vi "Auto_New.vi"() -> ()   [LabVIEW 2017]
uses:
  Control/Saurabh/prosucer_consumer_enum1.ctl
  <vilib>/Utility/error.llb/DialogType.ctl
  <vilib>/addons/database/Connection.llb/DB Tools Open Connec (String).vi
  Global/DATA LOG.vi
  Global/Global 1.vi
  <vilib>/addons/database/NI_Database_API.lvlib
panel:
  out "SHIFT":string
  in  "BARCODE RECIPE":string(combo)
  out "PLC COM.":bool
  out "SHIFT_DATA":string[](array[string])
  out "stop":bool
  out "error out 2":errorcluster
  out "Shift 4":i32
  out "Time Stamp Out":timestamp[](array[timestamp]) format="%<%X>T"
  out "Time Stamp Out 4":timestamp[](array[timestamp]) format="%<%X>T"
  out "Shift_change":bool
  out "appended array":string[][](array[string])
  out "SHIFT_DATA 2":string[](array[string])
  in  "error in (no error)":errorcluster
  in  "Tab Control":enum32{"Screen 1", "Screen 2", "Daignostic"}(tab)
  out "OP 50":bool
  out "OP 40":bool
  out "OP 30":bool
  out "OP - 50":T1 {"RH Motor Screw" format="%#.2g N-m"; "LH Motor Screw" format="%#.2g N-m"; "Nut Torque" format="%#.2g N-m"}
  out "OP - 40":T2 {"Stack Load" format="%.2f kg"; "Dispalcement" format="%#.2g mm"; "LH Screw" format="%#.2g N-m"; "RH Screw" format="%#.2g N-m"}
  out "OP - 30":T3 {"Shaft Press Load" format="%#.2g kg"; "Displacement" format="%#.2g mm"}
  in  "stop 2":bool
  out "OP - 10":T4 {"Leak Rate" format="%#.2g SCCM"}
  in  "SIMULATE INPUT":bool[](array[boolean])=[FALSE, FALSE, FALSE, FALSE]
  out "OP - 20":T5 {"Top Load" format="%#.2g kg"; "Top Displace" format="%#.2g mm"; "Bottom Load" format="%#.2g kg"; "Bottom Displace" format="%#.2g mm"}
  out "OP 10 & 20":bool
  out "OP - 60":T6 {"Screw 6" format="%#.2g N-m"; "Screw 5" format="%#.2g N-m"; "Screw 4" format="%#.2g N-m"; "Screw 3" format="%#.2g N-m"; "Screw 2" format="%#.2g N-m"; "Screw 1" format="%#.2g N-m"}
  out "OP - 70":T7 {"Full Open" format="%#.4g V"; "Full Close" format="%#.4g V"}
  out "OP - 110":cluster{"BARCODE":string}
  out "OP - 80":T8 {"Plug Press Load" format="%#.2f kg"}
  out "OP - 90":T9 {"Steam Leak" format="%#_g sccm"; "Seat Leak" format="%#_g LPM"}
  out "OP - 100":T10 {"Response Time REV" format="%#_g msec"; "Response time FWD" format="%#_g msec"; "Motor Full Open" format="%#.2f V"; "Motor Start Back" format="%#.2f V"; "Motor Full Close" format="%#.2f V"; "Motor Start Of Close" format="%#.2f V"; "Motor Peak" format="%#.2f A"; "Sensor O/P Full Close" format="%#.2f V"; "Sensor O/P Start Of Close" format="%#.2f V"; "Sensor O/P Open" format="%#.2f V"}
  out "OP 60":bool
  out "OP 70 & 80":bool
  out "OP 90 -100 - 110":bool
  out "OP110 STATUS":dbl[](array[numeric])
  out "SCAN OP110":string[](array[string])
  out "OP100 STATUS":dbl[](array[numeric])
  out "SCAN OP100":string[](array[string])
  out "OP50 STATUS":dbl[](array[numeric])
  out "SCAN OP50":string[](array[string])
  out "OP90 STATUS":dbl[](array[numeric])
  out "SCAN OP90":string[](array[string])
  out "OP80 STATUS":dbl[](array[numeric])
  out "SCAN OP80":string[](array[string])
  out "OP70 STATUS":dbl[](array[numeric])
  out "SCAN OP70":string[](array[string])
  out "OP60 STATUS":dbl[](array[numeric])
  out "SCAN OP60":string[](array[string])
  out "OP40 STATUS":dbl[](array[numeric])
  out "SCAN OP40":string[](array[string])
  out "OP30 STATUS":dbl[](array[numeric])
  out "SCAN OP30":string[](array[string])
  out "OP20 STATUS":dbl[](array[numeric])
  out "SCAN OP20":string[](array[string])
  out "OP10 STATUS":dbl[](array[numeric])
  out "SCAN OP10":string[](array[string])
  # "Op10 20\nOp30\nOp 40\nOp50\nOp60\nOp70-80\nOp 90-100-110"
  # "SENSOR MIN VLTG"
  # "OP - 50"
  # "OP - 40"
  # "OP - 30"
  # "OP - 10"
  # "OP - 20"
  # "OP - 60"
  # "OP - 70"
  # "OP - 110"
  # "OP - 80"
  # "OP - 90"
  # "OP - 100"
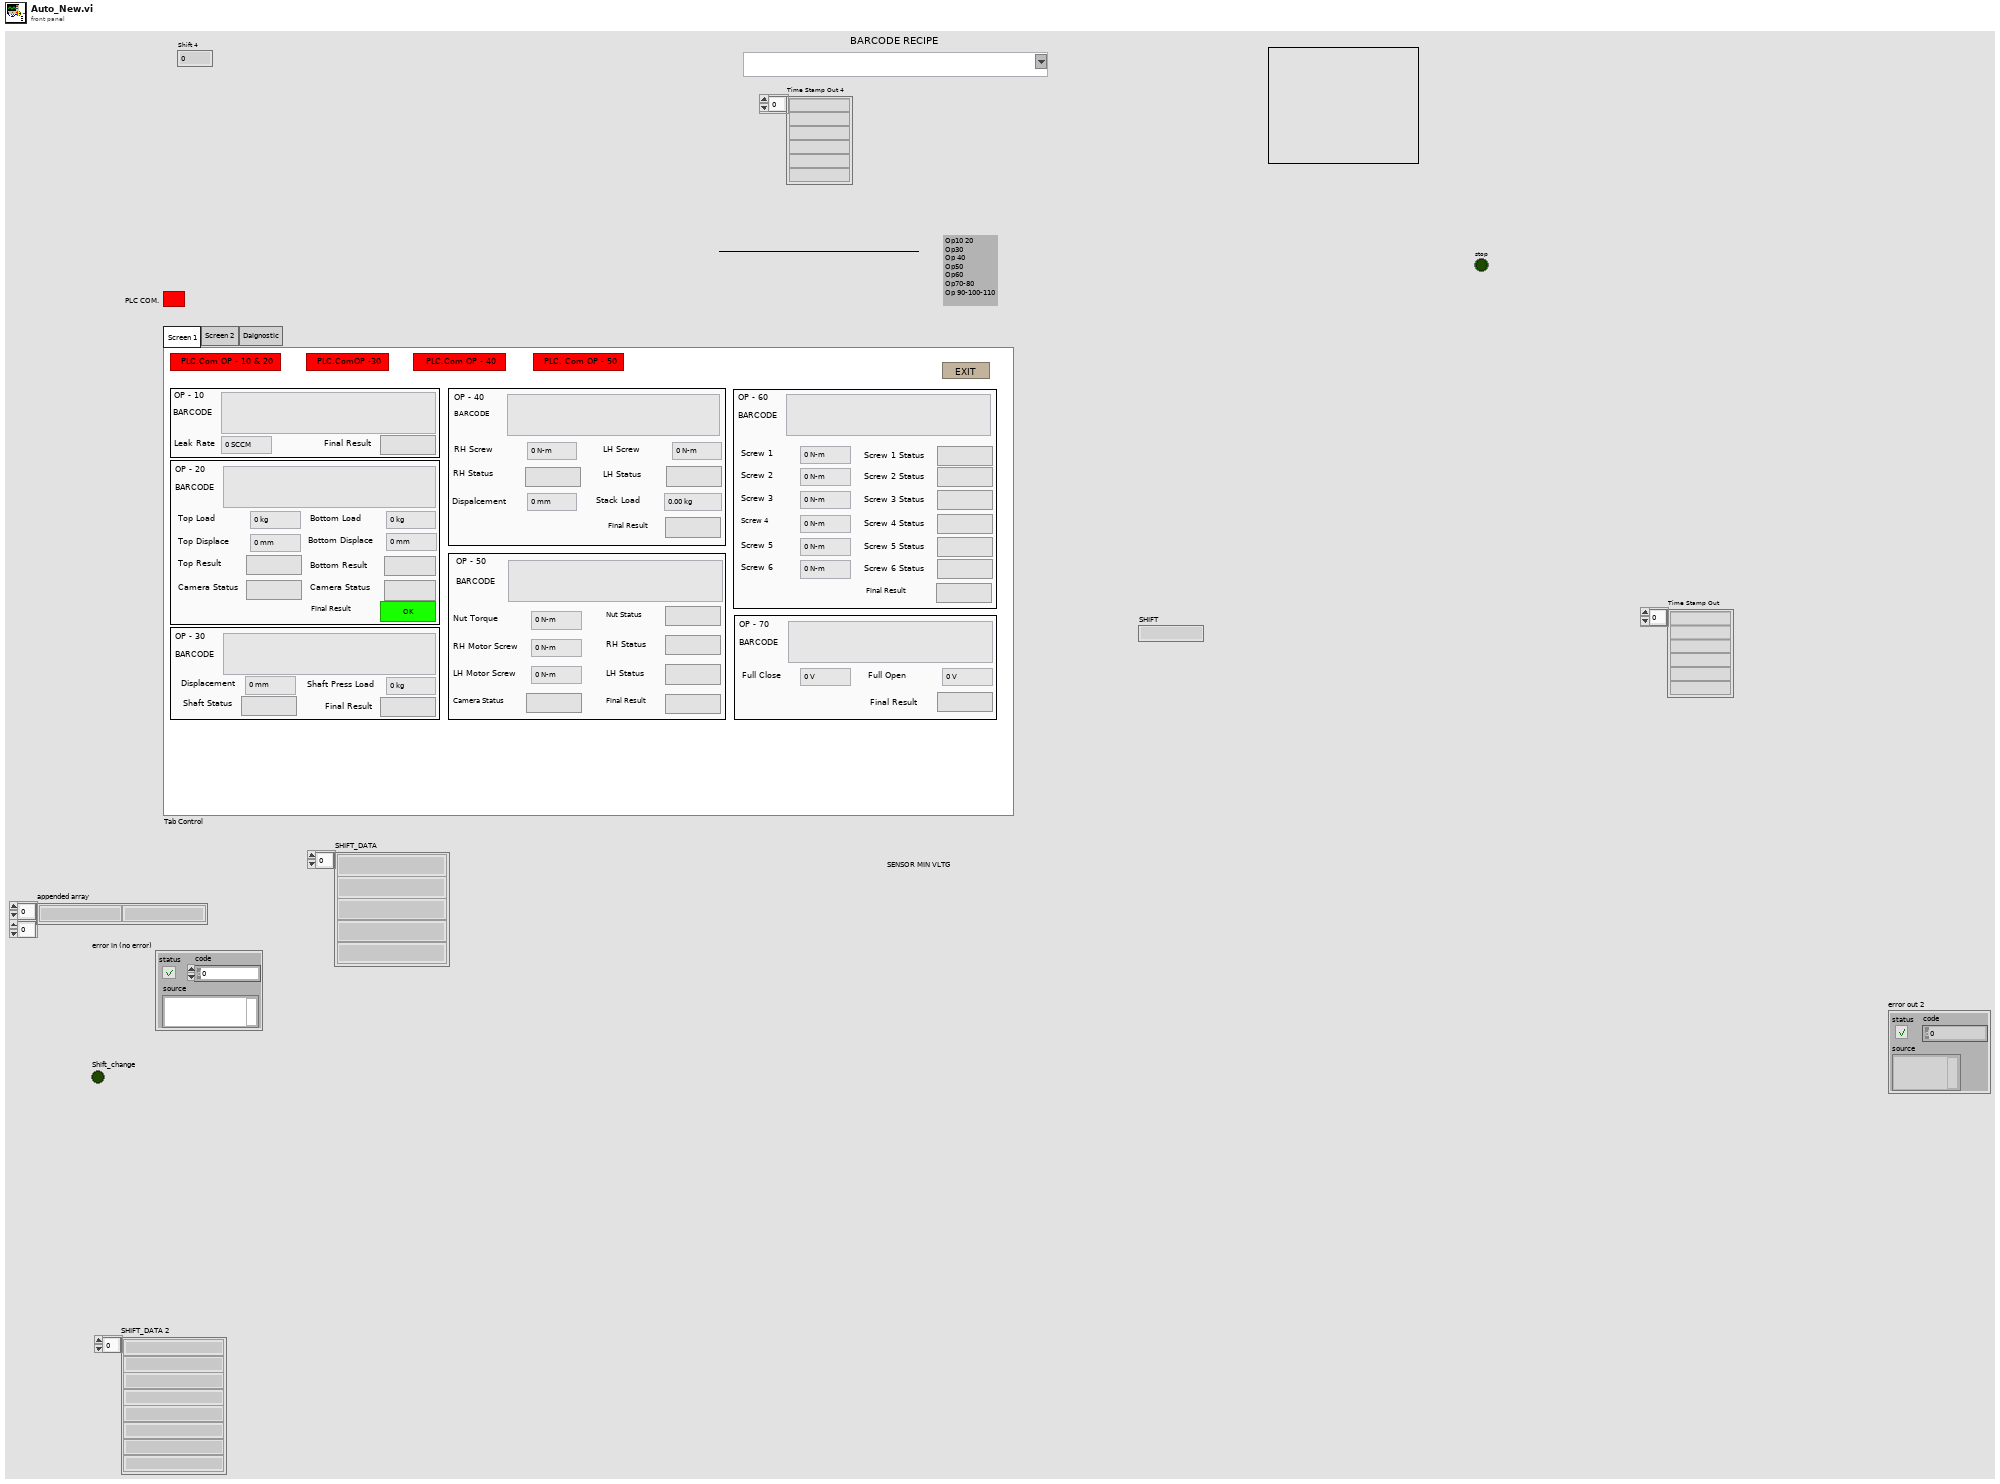
[diagram p1: front panel]
types:
  T1 = cluster{"BARCODE":string, "Nut Torque":dbl, "LH Motor Screw":dbl, "LH Status":bool, "RH Status":bool, "RH Motor Screw":dbl, "Final Result":bool, "Nut Status":bool, "Camera Status":bool}
  T2 = cluster{"BARCODE":string, "RH Screw":dbl, "LH Screw ":dbl, "RH Status":bool, "LH Status":bool, "Dispalcement ":dbl, "Stack Load ":dbl, "Final Result":bool}
  T3 = cluster{"BARCODE":string, "Displacement":dbl, "Shaft Press Load":dbl, "Shaft Status":bool, "Final Result":bool}
  T4 = cluster{"BARCODE":string, "Leak Rate":dbl, "Final Result":bool}
  T5 = cluster{"BARCODE":string, "Bottom Displace":dbl, "Bottom Load":dbl, "Camera Status":bool, "Bottom Result":bool, "Top Displace":dbl, "Top Load ":dbl, "Camera Status":bool, "Top Result":bool, "Final Result":bool}
  T6 = cluster{"BARCODE":string, "Screw 1":dbl, "Screw 2":dbl, "Screw 1 Status":bool, "Screw 2 Status":bool, "Screw 3":dbl, "Final Result":bool, "Screw 3 Status":bool, "Screw 4":dbl, "Screw 5":dbl, "Screw 4 Status":bool, "Screw 5 Status":bool, "Screw 6":dbl, "Screw 6 Status":bool}
  T7 = cluster{"BARCODE":string, "Full Close":dbl, "Full Open":dbl, "Final Result":bool}
  T8 = cluster{"BARCODE":string, "Plug Press Load":dbl, "Final Result":bool, "Loctite Status":bool}
  T9 = cluster{"BARCODE":string, "Seat Leak":dbl, "Seat Status":bool, "Steam Leak":dbl, "Final Result":bool}
  T10 = cluster{"BARCODE":string, "Sensor O/P Open":dbl, "Sensor O/P Start Of Close":dbl, "Final Result":bool, "Sensor O/P Full Close":dbl, "Motor Peak":dbl, "Motor Start Of Close":dbl, "Motor Full Close":dbl, "Motor Start Back":dbl, "Motor Full Open":dbl, "Response time FWD":dbl, "Response Time REV":dbl}
  T11 = cluster{"OP - 10":cluster{"BARCODE":string, "LEAK RATE":dbl, "RESULT":bool}, "OP - 30":cluster{"BARCODE":string, "Displacement":dbl, "Load":dbl, "Middle Gear Shaft Status":bool, "Final Result":bool}, "OP - 60":cluster{"BARCODE":string, "Screw 1 Data":dbl, "Screw 2 data":dbl, "Screw 1 Status":bool, "Screw 2 Status":bool, "Screw3 Data":dbl, "Final Result":bool, "Screw3 Status":bool, "Screw4 Data":dbl, "Screw5 Data":dbl, "Screw4 Status":bool, "Screw5 Status":bool, "Screw6 Data":dbl, "Screw6 Status":bool}, "OP - 70":cluster{"BARCODE":string, "Sensor MIN Vltg":dbl, "Sensor MAX Vltg":dbl, "Final Result":bool}, "OP - 80":cluster{"BARCODE":string, "Load":dbl, "Final Result":bool, "Dispensing":bool}, "OP - 90":cluster{"BARCODE":string, "Seat LT Data":dbl, "Seat Status":bool, "Steam LT Data":dbl, "Final Result":bool}, "OP - 110":cluster{"BARCODE":string}, "OP - 20":cluster{"BARCODE":string, "Bottom Displace":dbl, "Bottom Load":dbl, "Camera Status":bool, "Bottom Result":bool, "Top Displace":dbl, "Top Load ":dbl, "Camera Status":bool, "Top Result":bool, "Final Result":bool}, "OP - 40":cluster{"BARCODE":string, "RH Screw":dbl, "LH Screw ":dbl, "RH Status":bool, "LH Status":bool, "Dispalcement ":dbl, "Stack Load ":dbl, "Final Result":bool}, "OP - 50":cluster{"BARCODE":string, "Nut Torque":dbl, "LH Motor Screw":dbl, "LH Status":bool, "RH Status":bool, "RH Motor Screw":dbl, "Final Result":bool, "Nut Status":bool, "Camera Status":bool}, "OP - 100":cluster{"BARCODE":string, "Sensor O/P Open":dbl, "Sensor O/P Start Of Close":dbl, "Final Result":bool, "Sensor O/P Full Close":dbl, "Motor Peak":dbl, "Motor Start Of Close":dbl, "Motor Full Close":dbl, "Motor Start Back":dbl, "Motor Full Open":dbl, "Response time FWD":dbl, "Response Time REV":dbl}}
  T12 = typedef "prosucer_consumer_enum1.ctl" = enum16{"-1", "SCAN1", "SCAN2", "SCAN3", "SCAN4", "SCAN5", "SCAN6", "SCAN7", "SCAN8", "SCAN9", "SCAN10", "SCAN11", "STOP", "DATALOG1", "DATALOG2", "DATALOG3", "DATALOG4", "DATALOG5", "DATALOG6", "DATALOG7", "DATALOG8", "DATALOG9", "DATALOG10", "DATALOG11", "CYCLE_START1", "CYCLE_START2", "CYCLE_START3", "CYCLE_START4", "BARCODE RECIPE", "EMERGENCY STOP"}
  T13 = typedef "NI_Database_API.lvlib/Conn ObjectReference.ctl" = refnum<k1>
  T14 = typedef "DialogType.ctl" = u16
  T15 = cluster{"trimmed string":string, "SHIFT":string, "date/time string":string, string, "Input 2":string}
  T16 = cluster{"SHIFT":string, "date/time string":string, "Input 2":string, string}
  T17 = cluster{"date/time string":string, "Input 2":string, "Input 2":string, "Input 2":string, "Input 2":string, "Input 2":string, "Input 2":string, "Input 2":string, "Input 2":string, "Input 2":string, "Input 2":string}
  T18 = cluster{"date/time string":string, "SHIFT":string, "Input 2":string, "Input 2":string, "Input 2":string, "Input 2":string, "Input 2":string, "Input 2":string, "Input 2":string, "Input 2":string, "Input 2":string, "Input 2":string}
  T19 = cluster{"date/time string":string, "Input 2":string, "Input 2":string, "Input 2":string, "Input 2":string}
  T20 = cluster{"date/time string":string, "SHIFT":string, "Input 2":string, "Input 2":string, "Input 2":string, "Input 2":string}
  T21 = cluster{"date/time string":string, "Input 2":string, "Input 2":string, "Input 2":string, "Input 2":string, "Input 2":string, "Input 2":string, "Input 2":string, "Input 2":string}
  T22 = cluster{"date/time string":string, "SHIFT":string, "Input 2":string, "Input 2":string, "Input 2":string, "Input 2":string, "Input 2":string, "Input 2":string, "Input 2":string, "Input 2":string}
  T23 = cluster{"date/time string":string, "Input 2":string, "Input 2":string, "Input 2":string, "Input 2":string, "Input 2":string, "Input 2":string, "Input 2":string}
  T24 = cluster{"date/time string":string, "SHIFT":string, "Input 2":string, "Input 2":string, "Input 2":string, "Input 2":string, "Input 2":string, "Input 2":string}
  T25 = cluster{"date/time string":string, "Input 2":string, "Input 2":string, "Input 2":string, "Input 2":string, "Input 2":string, "Input 2":string, "Input 2":string, "Input 2":string, "Input 2":string, "Input 2":string, "Input 2":string, "Input 2":string, "Input 2":string}
  T26 = cluster{"date/time string":string, "SHIFT":string, "Input 2":string, "Input 2":string, "Input 2":string, "Input 2":string, "Input 2":string, "Input 2":string, "Input 2":string, "Input 2":string, "Input 2":string, "Input 2":string, "Input 2":string, "Input 2":string}
  T27 = cluster{"date/time string":string, "Input 2":string, "Input 2":string, "Input 2":string}
  T28 = cluster{"date/time string":string, "SHIFT":string, "Input 2":string, "Input 2":string, "Input 2":string}
  T29 = cluster{"date/time string":string, "Input 2":string, "Input 2":string, "Input 2":string, "Input 2":string, "Input 2":string, "Input 2":string, "Input 2":string, "Input 2":string, "Input 2":string, "Input 2":string, "Input 2":string, "Input 2":string}
  T30 = cluster{"BARCODE":string, "Seat LT Data":dbl, "Seat Status":bool, "Steam LT Data":dbl, "Final Result":bool}
  T31 = cluster{"BARCODE":string, "LEAK RATE":dbl, "RESULT":bool}
  T32 = cluster{"BARCODE":string, "Displacement":dbl, "Load":dbl, "Middle Gear Shaft Status":bool, "Final Result":bool}
  T33 = cluster{"BARCODE":string, "Screw 1 Data":dbl, "Screw 2 data":dbl, "Screw 1 Status":bool, "Screw 2 Status":bool, "Screw3 Data":dbl, "Final Result":bool, "Screw3 Status":bool, "Screw4 Data":dbl, "Screw5 Data":dbl, "Screw4 Status":bool, "Screw5 Status":bool, "Screw6 Data":dbl, "Screw6 Status":bool}
  T34 = cluster{"BARCODE":string, "Sensor MIN Vltg":dbl, "Sensor MAX Vltg":dbl, "Final Result":bool}
  T35 = cluster{"BARCODE":string, "Load":dbl, "Final Result":bool, "Dispensing":bool}
  T36 = enum32{"invalid app kind", "Development System", "Run Time System", "Student Edition", "Embedded LabVIEW", "Evaluation", "Custom"}
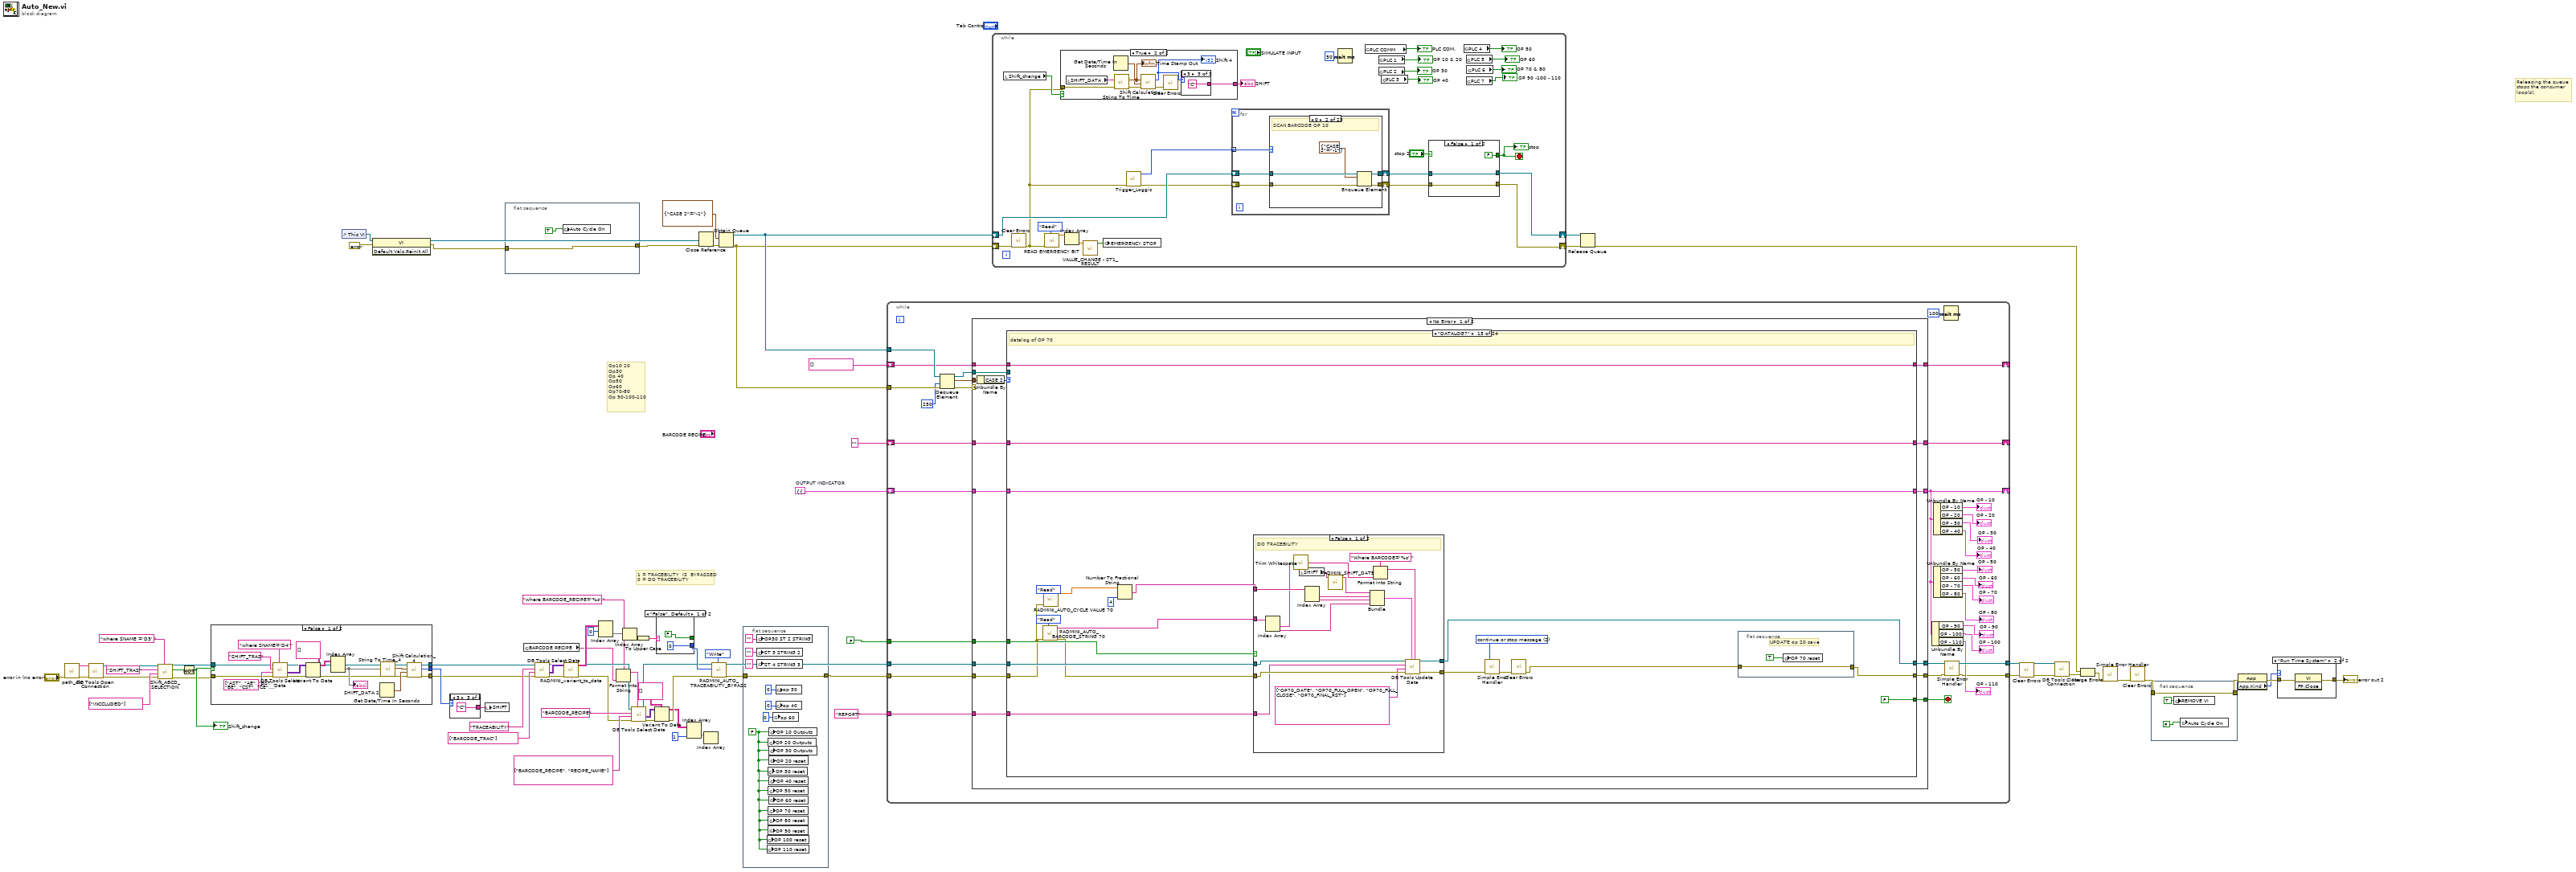
[diagram p0: block diagram]
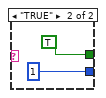
[diagram p2: hidden frame]
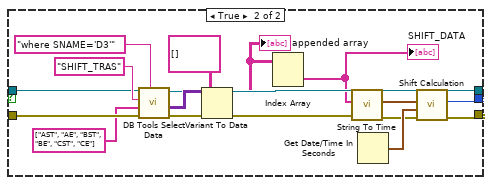
[diagram p3: hidden frame]
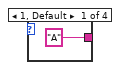
[diagram p4: hidden frame]
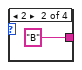
[diagram p5: hidden frame]
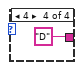
[diagram p6: hidden frame]
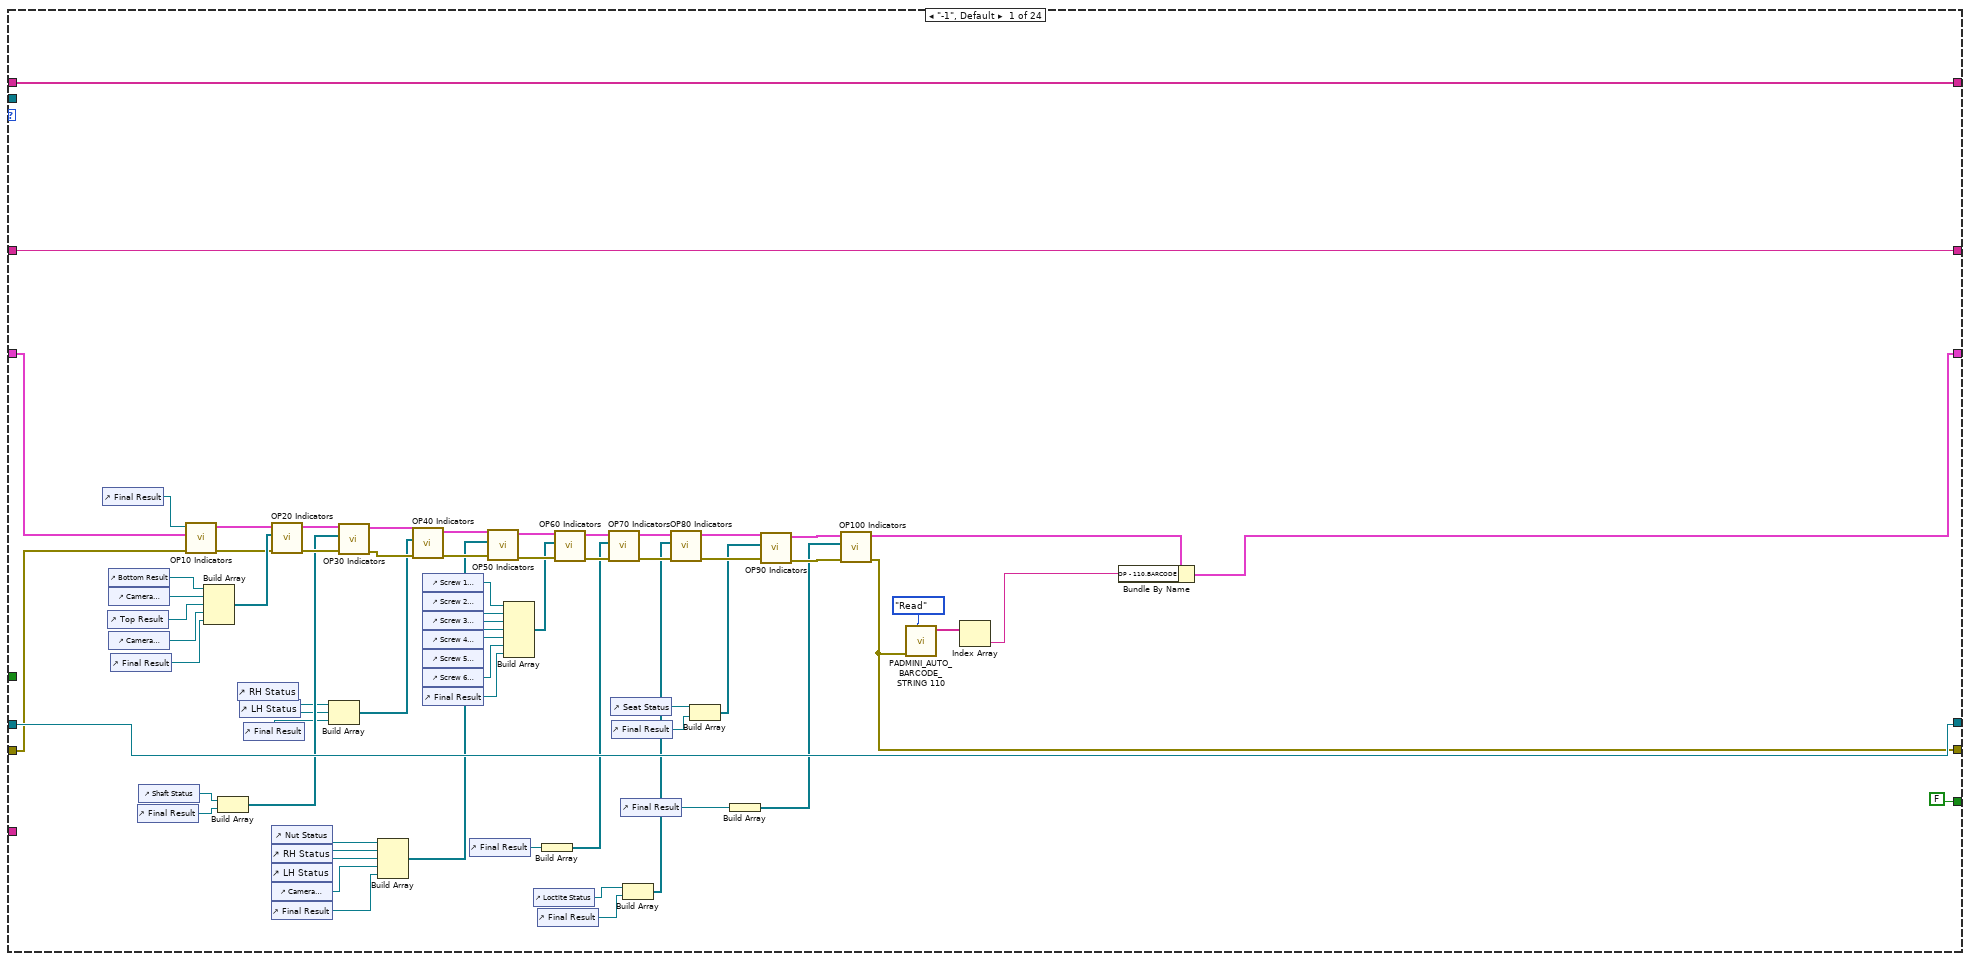
[diagram p7: hidden frame]
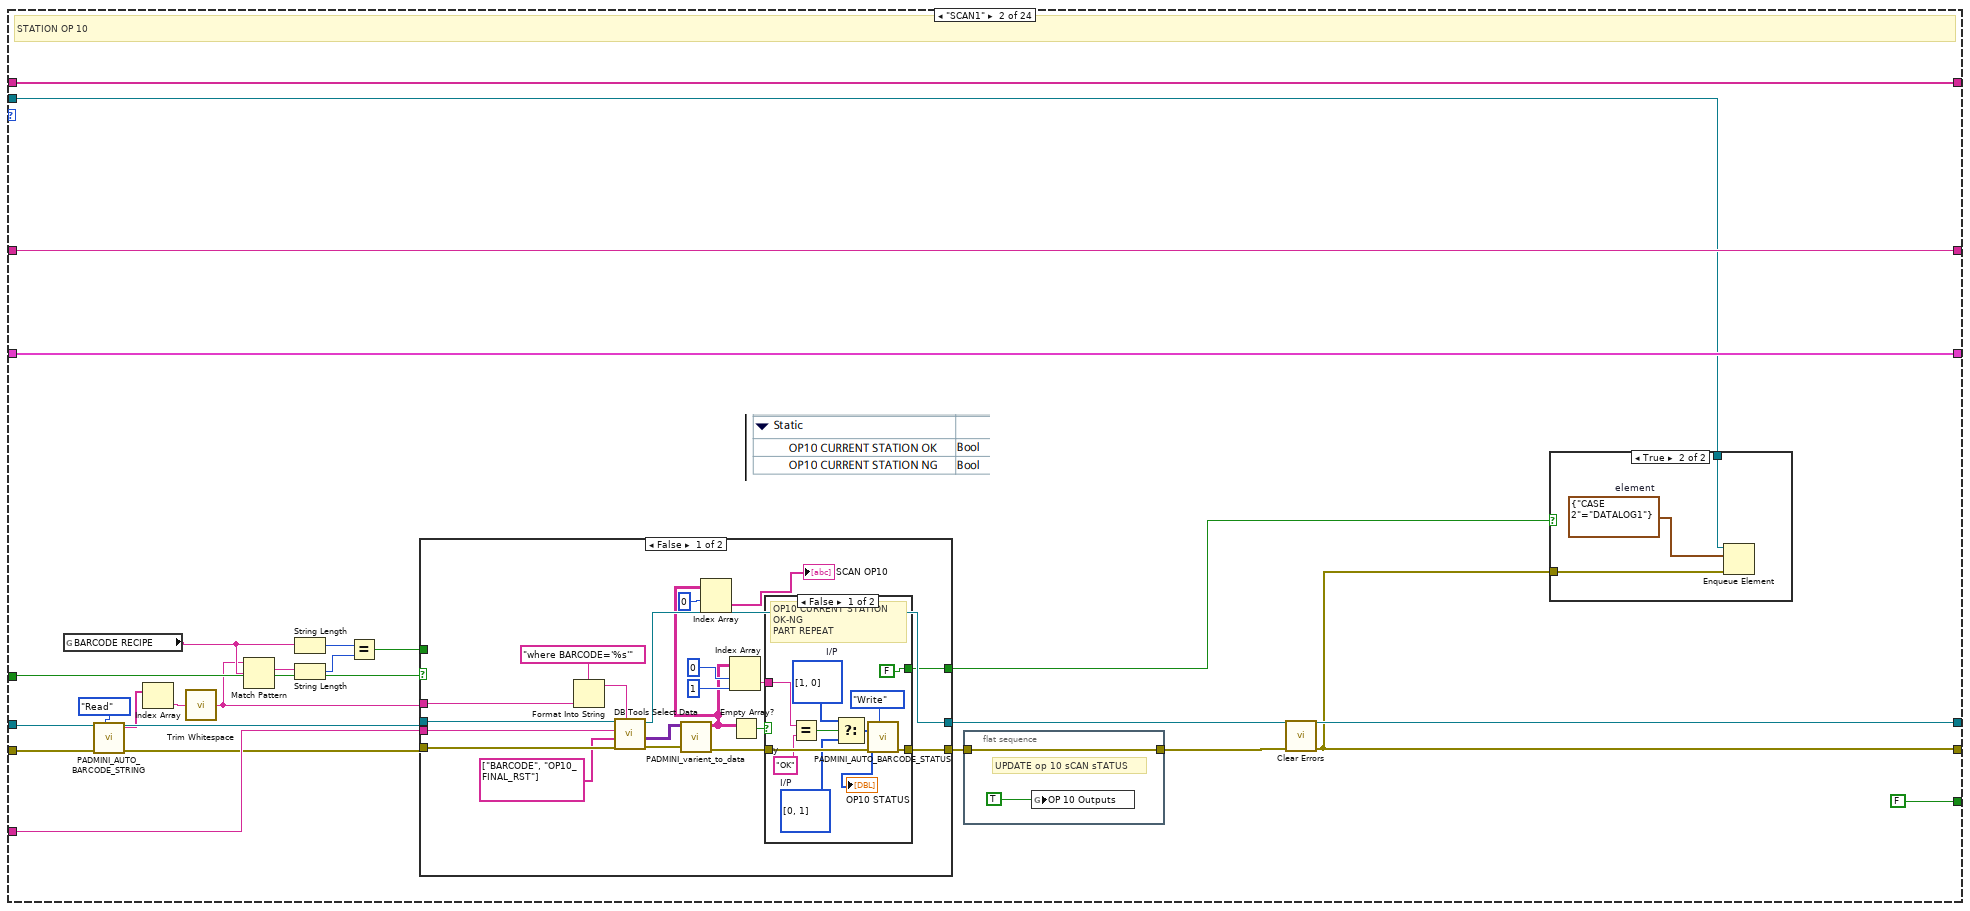
[diagram p8: hidden frame]
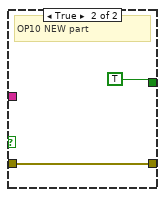
[diagram p10: hidden frame]
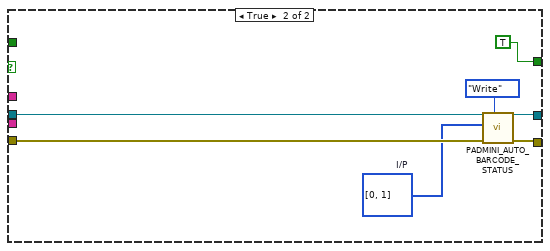
[diagram p11: hidden frame]
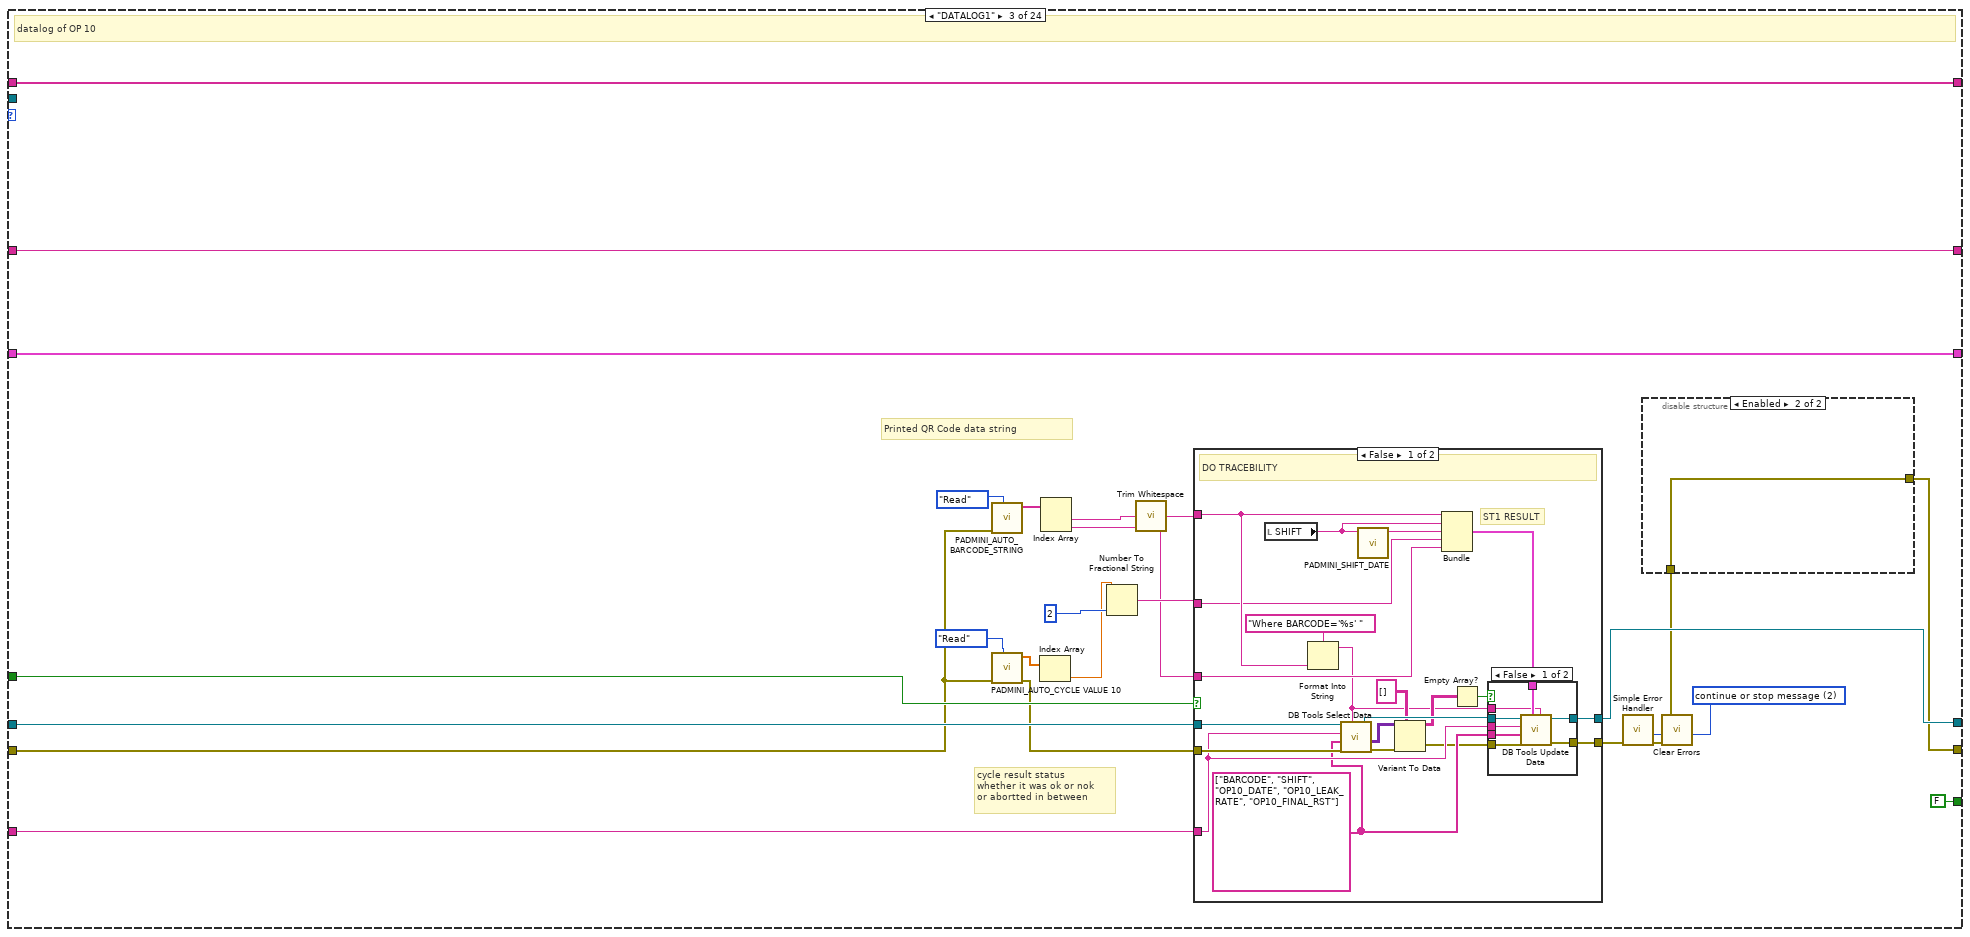
[diagram p12: hidden frame]
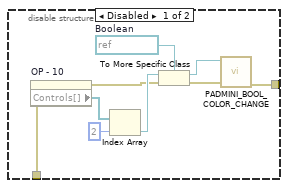
[diagram p13: hidden frame]
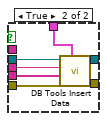
[diagram p14: hidden frame]
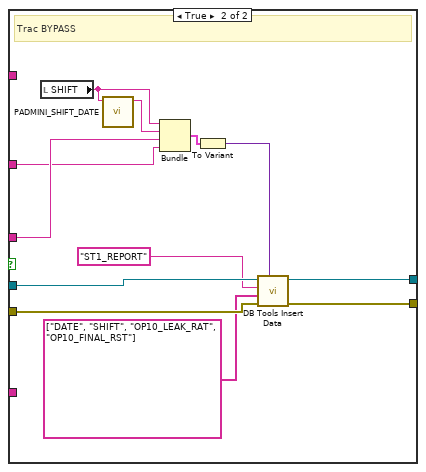
[diagram p15: hidden frame]
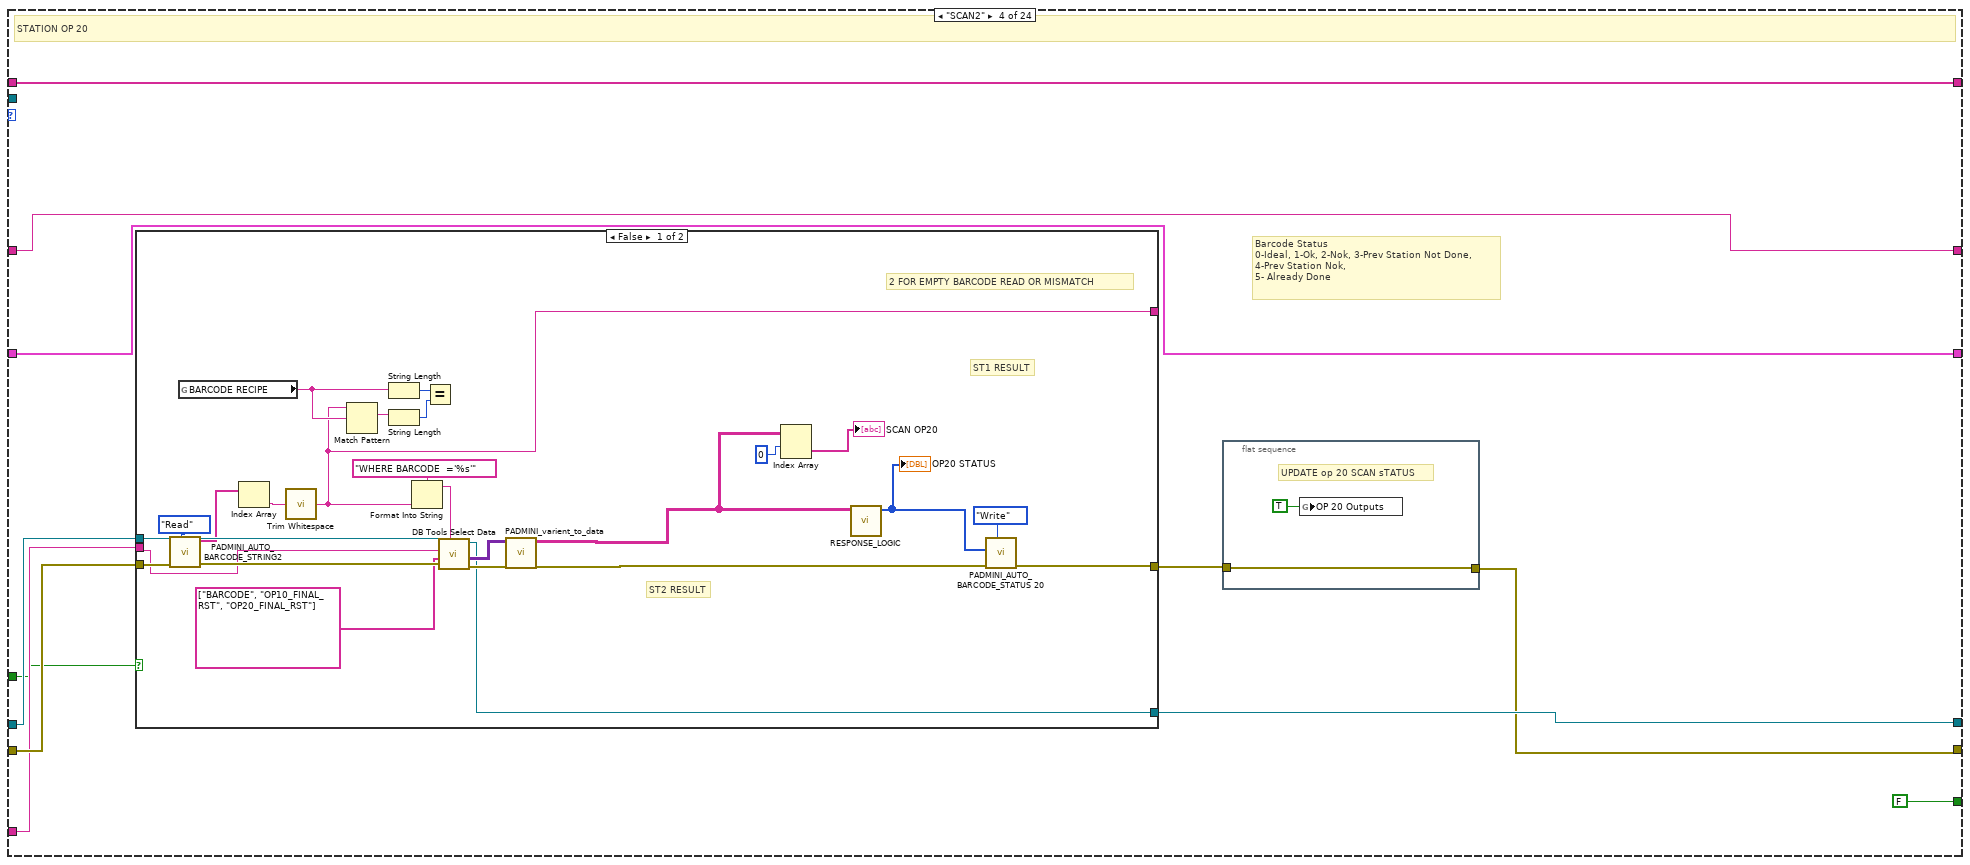
[diagram p16: hidden frame]
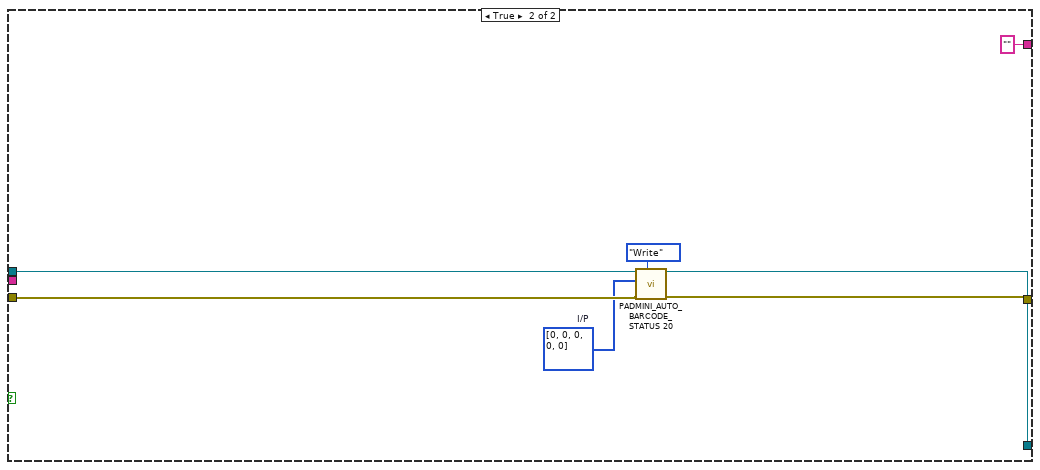
[diagram p17: hidden frame]
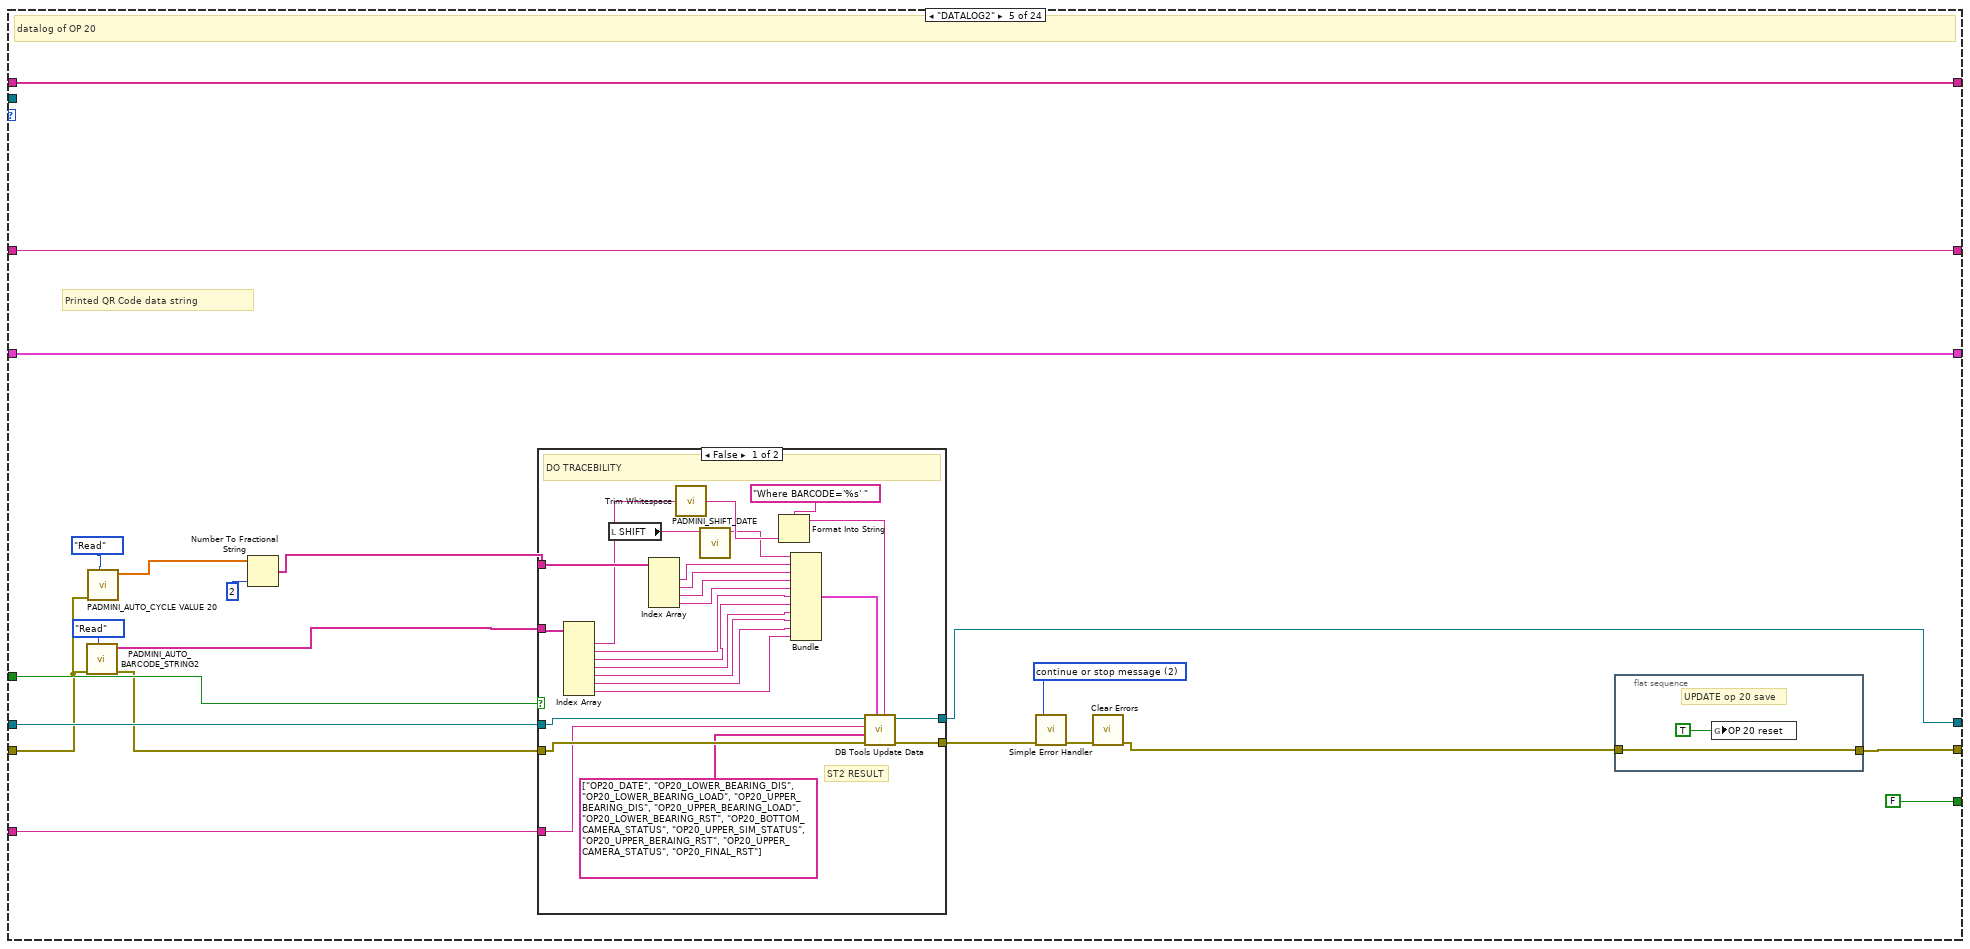
[diagram p18: hidden frame]
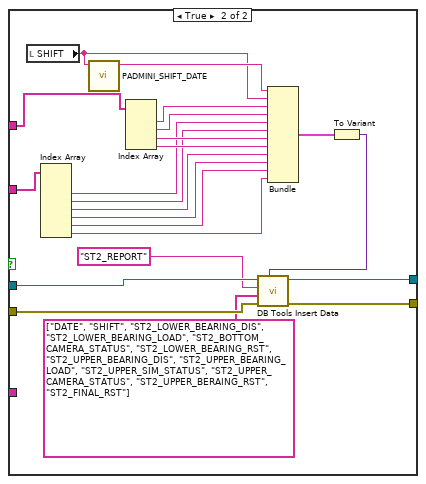
[diagram p19: hidden frame]
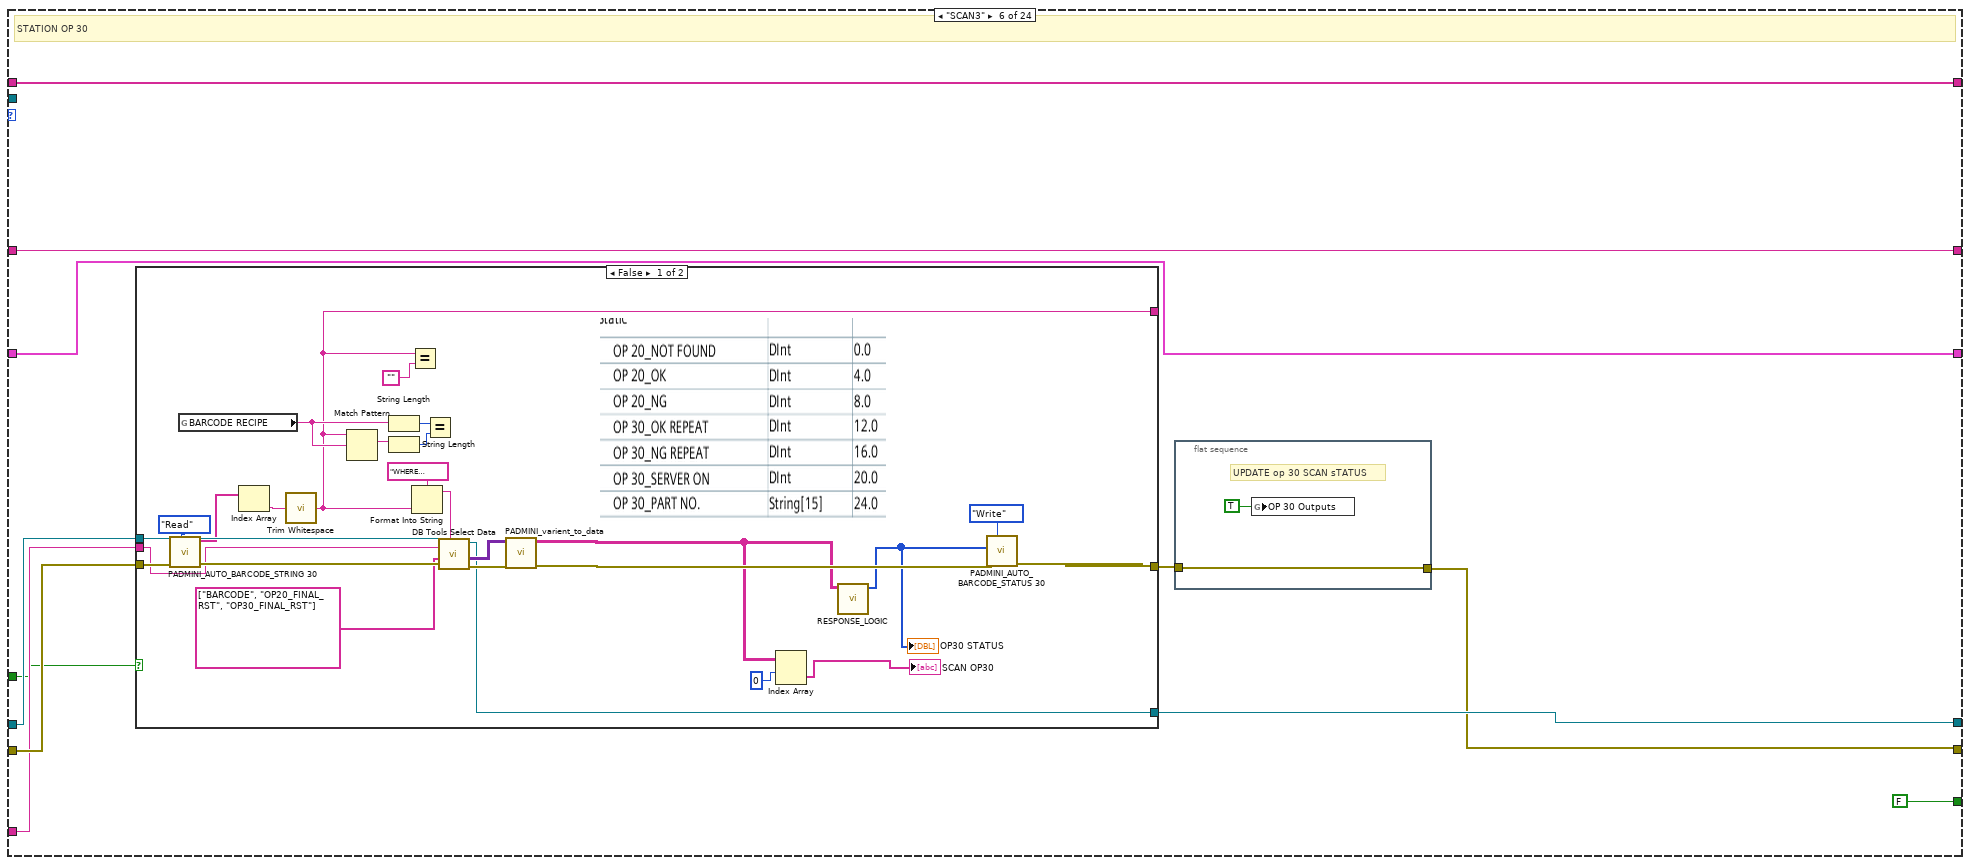
[diagram p20: hidden frame]
diagram:
  w1 = T11 {"OP - 10"={"BARCODE"="", "LEAK RATE"=0.0, "RESULT"=FALSE}, "OP - 30"={"BARCODE"="", "Displacement"=0.0, "Load"=0.0, "Middle Gear Shaft Status"=FALSE, "Final Result"=FALSE}, "OP - 60"={"BARCODE"="", "Screw 1 Data"=0.0, "Screw 2 data"=0.0, "Screw 1 Status"=FALSE, "Screw 2 Status"=FALSE, "Screw3 Data"=0.0, "Final Result"=FALSE, "Screw3 Status"=FALSE, "Screw4 Data"=0.0, "Screw5 Data"=0.0, "Screw4 Status"=FALSE, "Screw5 Status"=FALSE, "Screw6 Data"=0.0, "Screw6 Status"=FALSE}, "OP - 70"={"BARCODE"="", "Sensor MIN Vltg"=0.0, "Sensor MAX Vltg"=0.0, "Final Result"=FALSE}, "OP - 80"={"BARCODE"="", "Load"=0.0, "Final Result"=FALSE, "Dispensing"=FALSE}, "OP - 90"={"BARCODE"="", "Seat LT Data"=0.0, "Seat Status"=FALSE, "Steam LT Data"=0.0, "Final Result"=FALSE}, "OP - 110"={"BARCODE"=""}, "OP - 20"={"BARCODE"="", "Bottom Displace"=0.0, "Bottom Load"=0.0, "Camera Status"=FALSE, "Bottom Result"=TRUE, "Top Displace"=0.0, "Top Load "=0.0, "Camera Status"=FALSE, "Top Result"=FALSE, "Final Result"=FALSE}, "OP - 40"={"BARCODE"="", "RH Screw"=0.0, "LH Screw "=0.0, "RH Status"=FALSE, "LH Status"=FALSE, "Dispalcement "=0.0, "Stack Load "=0.0, "Final Result"=FALSE}, "OP - 50"={"BARCODE"="", "Nut Torque"=0.0, "LH Motor Screw"=0.0, "LH Status"=FALSE, "RH Status"=FALSE, "RH Motor Screw"=0.0, "Final Result"=FALSE, "Nut Status"=FALSE, "Camera Status"=FALSE}, "OP - 100"={"BARCODE"="", "Sensor O/P Open"=0.0, "Sensor O/P Start Of Close"=0.0, "Final Result"=FALSE, "Sensor O/P Full Close"=0.0, "Motor Peak"=0.0, "Motor Start Of Close"=0.0, "Motor Full Close"=0.0, "Motor Start Back"=0.0, "Motor Full Open"=0.0, "Response time FWD"=0.0, "Response Time REV"=0.0}}  # OUTPUT INDICATOR
  # "Op10 20\nOp30\nOp 40\nOp50\nOp60\nOp70-80\nOp 90-100-110"
  # "1 = TRACEBILITY  IS  BYPASSED\n0 = DO TRACEBILITY"
  # "Releasing the queue stops the consumer loop(s)."
  n1 = call "path_db.vi"("error in"="error in (no error)") -> ("error out"=w48:errorcluster, "resulting string"=w69:string)  [unwired: 9 in]
  n2 = call-poly <vilib>:"DB Tools Open Connection.vi"("error in (no error)"=w48, "connection information"=w69) -> ("error out"=w47:errorcluster, "connection reference"=w41:T13)  [unwired: 6 in]
  n3 = call "Shift_ABCD_SELECTION.vi"("Where"="where SNAME ='D3' ", "error in (no error)"=w47, "Array"=string[] ["INCCLUDED"], "table"="SHIFT_TRAS", "Refnum in"=w41) -> ("error out"=w5:errorcluster, "Boolean"=w60:bool, "Refnum out"=w61:T13)  [unwired: 4 in]
  n4 = Not(x=w60) -> (.not. x?=w59:bool)
  "Shift_change" <- w59
  n5 = case shown="False" w59 {
    tunnel: [w74 w98] -> w65
    tunnel: w61 -> [w77 w96]
    tunnel: w5 -> [w76 w95]
    tunnel: [w75 w94] -> w30
    tunnel: [w73 w88] -> w29
    frame False {
      n6 = call <vilib>:"DB Tools Select Data.vi"("condition"="where SNAME='D4'", "error in (no error)"=w76, "columns"=string[] ["AST", "AE", "BST", "BE", "CST", "CE", "DST", "DE"], "table"="SHIFT_TRAS", "connection reference"=w77) -> ("error out"=w83:errorcluster, "data"=w87:variant[][], "connection reference out"=w75:T13)  [unwired: 1 in]
      n7 = Variant To Data(error in=w83, type=string[][] [], Variant=w87) -> (data=w80:string[][], error out=w73:errorcluster)
      n8 = Index Array(array=w80) -> (element=w79:string[])  [unwired: 2 in]
      "SHIFT_DATA 2" <- w79
      n9 = Get Date/Time In Seconds() -> (seconds since 1Jan1904=w82:timestamp)
      n10 = call "String To Time_4.vi"("String Array In"=w79) -> ("Time Stamp Out"=w78:timestamp[])  [unwired: 9 in, 1 out]
      n11 = call "Shift Calculation_4.vi"("Current Time"=w82, "Time Stamp Out"=w78) -> ("Shift"=w74:i32)  [unwired: 8 in, 1 out]
    }
    frame True {
      n12 = call <vilib>:"DB Tools Select Data.vi"("condition"="where SNAME='D3'", "error in (no error)"=w95, "columns"=string[] ["AST", "AE", "BST", "BE", "CST", "CE"], "table"="SHIFT_TRAS", "connection reference"=w96) -> ("error out"=w100:errorcluster, "data"=w104:variant[][], "connection reference out"=w94:T13)  [unwired: 1 in]
      n13 = Variant To Data(error in=w100, type=string[][] [], Variant=w104) -> (data=w92:string[][], error out=w90:errorcluster)
      "appended array" <- w92
      n14 = Index Array(array=w92) -> (element=w91:string[])  [unwired: 2 in]
      "SHIFT_DATA" <- w91
      n15 = call "String To Time.vi"("error in (no error)"=w90, "String Array In"=w91) -> ("error out"=w89:errorcluster, "Time Stamp Out"=w97:timestamp[])  [unwired: 8 in]
      n16 = Get Date/Time In Seconds() -> (seconds since 1Jan1904=w99:timestamp)
      n17 = call "Shift Calculation.vi"("error in (no error)"=w89, "Current Time"=w99, "Time Stamp Out"=w97) -> ("error out"=w88:errorcluster, "Shift"=w98:i32)  [unwired: 7 in]
    }
  }
  n18 = control-ref of="This VI"() -> (w45:refnum<vi>)
  n19 = invoke class="VI" method="Default Vals.Reinit All"(reference=w45, error in=errorcluster {"status"=FALSE, "code"=0, "source"=""} ("error in (no error)")) -> (reference out=w44:refnum<vi>, error out=w2:errorcluster)  [unwired: 1 in, 1 out]
  n20 = case shown="3" w65 {
    tunnel: ["A" "B" "C" "D"] -> w58
    frame 1, Default {
    }
    frame 2 {
    }
    frame 3 {
    }
    frame 4 {
    }
  }
  n21 = local write "SHIFT"(w58) -> ()
  n22 = flat-sequence {
    tunnel: [w110] -> w3
    tunnel: w2 -> [w110]
    frame #0 {
      n23 = global write "DATA LOG.vi" "Auto Cycle On"(TRUE) -> ()
    }
  }
  n24 = global read "Global 1.vi" "BARCODE RECIPE"() -> (w11:string)
  n25 = call <vilib>:"DB Tools Select Data.vi"("error in (no error)"=w29, "columns"=string[] ["BARCODE_TRAC"], "table"="TRACEABILITY", "connection reference"=w30) -> ("error out"=w39:errorcluster, "data"=w38:variant[][], "connection reference out"=w17:T13)  [unwired: 2 in]
  n26 = call "PADMINI_varient_to_data.vi"("error in (no error)"=w39, "data"=w38) -> ("error out"=w15:errorcluster, "Array"=w37:string[][])  [unwired: 8 in]
  n27 = Index Array(array=w37, index (row)=0 ("disabled index (col)")) -> (element=w36:string[])  [unwired: 1 in]
  n28 = Format Into String(format string="where BARCODE_RECIPE='%s' ", w11) -> (resulting string=w9:string)  [unwired: 2 in, 1 out]
  n29 = Index Array(array=w36) -> (element=w32:string)  [unwired: 1 in]
  n30 = call <vilib>:"DB Tools Select Data.vi"("condition"=w9, "error in (no error)"=w15, "columns"=string[] ["BARCODE_RECIPE", "RECIPE_NAME"], "table"="BARCODE_RECIPE", "connection reference"=w17) -> ("error out"=w19:errorcluster, "data"=w18:variant[][], "connection reference out"=w16:T13)  [unwired: 1 in]
  n31 = To Upper Case(1:w32) -> (0:w31:string)
  n32 = Variant To Data(error in=w19, type=string[][] [], Variant=w18) -> (data=w12:string[][], error out=w14:errorcluster)
  n33 = case shown="\"False\", Default" w31 {
    tunnel: [FALSE ("BARCODE TRACEABILITY") TRUE ("BARCODE TRACEABILITY")] -> _
    tunnel: [0 1] -> w27
    frame "False", Default {
    }
    frame "TRUE" {
    }
  }
  n34 = Index Array(array=w12, index (col)=1 ("disabled index (col)")) -> (element=w7:string[])  [unwired: 1 in]
  n35 = Close Reference(reference=w44, error in (no error)=w3) -> (error out=w42:errorcluster)
  n36 = Index Array(array=w7) -> ()  [unwired: 1 in, 1 out]
  n37 = call "PADMINI_AUTO_TRACEABILITY_BYPASS.vi"("Enum"=enum16{"Read", "Write"}."Write", "error in (no error)"=w14, "I/P"=w27) -> ("error out"=w25:errorcluster)  [unwired: 7 in, 1 out]
  n38 = Obtain Queue(element data type=cluster{"CASE 2":T12} {"CASE 2"=enum."-1"}, error in (no error)=w42) -> (queue out=w70:refnum<queue>, error out=w22:errorcluster)  [unwired: 3 in, 1 out]
  n39 = flat-sequence {
    tunnel: w25 -> [w119]
    tunnel: [w119] -> w24
    frame #0 {
      w115 = FALSE
      n40 = global write "DATA LOG.vi" "OP30 ST 2 STRING"("" ("OP30 ST 2 STRING")) -> ()
      n41 = global write "DATA LOG.vi" "ST 3 STRING 2"("" ("ST 3 STRING 2")) -> ()
      n42 = global write "DATA LOG.vi" "ST 4 STRING 3"("" ("ST 4 STRING 3")) -> ()
      n43 = global write "DATA LOG.vi" "OP 100 reset"(w115) -> ()
      n44 = global write "DATA LOG.vi" "OP 110 reset"(w115) -> ()
      n45 = global write "DATA LOG.vi" "OP 30 reset"(w115) -> ()
      n46 = global write "DATA LOG.vi" "OP 20 Outputs"(w115) -> ()
      n47 = global write "DATA LOG.vi" "OP 50 reset"(w115) -> ()
      n48 = global write "DATA LOG.vi" "OP 70 reset"(w115) -> ()
      n49 = global write "DATA LOG.vi" "OP 80 reset"(w115) -> ()
      n50 = global write "DATA LOG.vi" "OP 90 reset"(w115) -> ()
      n51 = global write "DATA LOG.vi" "OP 10 Outputs"(w115) -> ()
      n52 = global write "DATA LOG.vi" "OP 30 Outputs"(w115) -> ()
      n53 = global write "DATA LOG.vi" "OP 20 reset"(w115) -> ()
      n54 = global write "DATA LOG.vi" "OP 40 reset"(w115) -> ()
      n55 = global write "DATA LOG.vi" "OP 60 reset"(w115) -> ()
      n56 = global write "DATA LOG.vi" "op 60"(0 ("op 30")) -> ()
      n57 = global write "DATA LOG.vi" "op 30"(0 ("op 30")) -> ()
      n58 = global write "DATA LOG.vi" "op 40"(0 ("op 30")) -> ()
    }
  }
  n59 = while {
    tunnel: w70 -> [w154]
    tunnel: w22 -> [w150]
    tunnel: w24 -> [w149]
    tunnel: w16 -> [w148]
    tunnel: [w123] -> w68
    tunnel: [w147] -> w67
    tunnel: FALSE -> [w146]
    tunnel: "REPORT" -> [w145]
    shift-right: [w143] -> _
    shift-left: string[] [] -> [w144]
    shift-right: [w142] -> _
    shift-left: "" ("trimmed string") -> [w141]
    shift-right: [w130] -> _
    shift-left: w1 -> [w139]
    stop <- w151 stop-if-true
    n60 = Dequeue Element(queue=w154, timeout in ms (-1)=250, error in (no error)=w150) -> (queue out=w126:refnum<queue>, element=w152:cluster{"CASE 2":T12}, error out=w153:errorcluster)  [unwired: 1 out]
    n61 = case shown="No Error" w153 {
      tunnel: w152 -> [w170 _]
      tunnel: [w166 TRUE] -> w151
      tunnel: w149 -> [w167 w1404]
      tunnel: w148 -> [w168 w1403]
      tunnel: [w164 w1404] -> w124
      tunnel: [w165 w1403] -> w147
      tunnel: w146 -> [w163 _]
      tunnel: w145 -> [w162 _]
      tunnel: w144 -> [w161 w1402]
      tunnel: [w160 w1402] -> w143
      tunnel: [w159 w1401] -> w142
      tunnel: w141 -> [w158 w1401]
      tunnel: w139 -> [w157 w1400]
      tunnel: [w156 w1400] -> w130
      tunnel: w126 -> [w155 _]
      frame No Error {
        n62 = Unbundle By Name(w170) -> ("CASE 2"=w169:T12)
        n63 = case shown="\"DATALOG7\"" w169 {
          tunnel: w168 -> [w237 w261 w329 w399 w452 w513 w567 w616 w665 w722 w771 w825 w874 w940 w989 w1036 w1085 w1132 w1181 w1230 w1270 w1329 w1387 w1395]
          tunnel: w167 -> [w234 w257 w306 w398 w439 w512 w553 w615 w651 w721 w758 w824 w860 w939 w975 w1035 w1071 w1131 w1167 w1229 w1269 w1311 w1386 w1397]
          tunnel: [FALSE FALSE FALSE FALSE FALSE FALSE FALSE FALSE FALSE FALSE FALSE FALSE FALSE FALSE FALSE FALSE FALSE FALSE FALSE FALSE FALSE FALSE FALSE TRUE] -> w166
          tunnel: [w237 w259 w326 w396 w449 w510 w564 w613 w662 w719 w768 w822 w871 w937 w986 w1033 w1082 w1129 w1178 w1227 w1267 w1326 w1387 w1394] -> w165
          tunnel: [w171 w239 w325 w393 w434 w507 w548 w610 w646 w716 w753 w819 w855 w934 w970 w1030 w1066 w1126 w1162 w1224 w1264 w1310 w1386 w1396] -> w164
          tunnel: w163 -> [_ w254 w328 w395 w451 w509 w566 w612 w664 w718 w770 w821 w873 w936 w988 w1032 w1084 w1128 w1180 w1226 w1266 w1328 _ _]
          tunnel: w162 -> [_ w260 w327 w397 w450 w511 w565 w614 w663 w720 w769 w823 w872 w938 w987 w1034 w1083 w1130 w1179 w1228 w1268 w1327 _ _]
          tunnel: w161 -> [w236 w258 w322 w390 w448 w505 w563 w608 w661 w714 w767 w817 w870 w932 w985 w1028 w1081 w1124 w1177 w1222 w1262 w1325 w1384 w1398]
          tunnel: [w236 w258 w322 w390 w448 w505 w563 w608 w661 w714 w767 w817 w870 w932 w985 w1028 w1081 w1124 w1177 w1222 w1262 w1325 w1384 w1398] -> w160
          tunnel: [w235 w253 w318 w391 w444 w504 w559 w607 w657 w713 w763 w816 w866 w931 w981 w1027 w1077 w1123 w1173 w1221 w1261 w1321 w1383 w1389] -> w159
          tunnel: w158 -> [w235 w253 w318 w391 w444 w504 w559 w607 w657 w713 w763 w816 w866 w931 w981 w1027 w1077 w1123 w1173 w1221 w1261 w1321 w1383 w1389]
          tunnel: w157 -> [w233 w247 w316 w389 w433 w503 w557 w606 w655 w712 w752 w815 w864 w930 w979 w1026 w1075 w1122 w1171 w1220 w1260 w1319 w1382 w1388]
          tunnel: [w175 w247 w316 w389 w433 w503 w557 w606 w655 w712 w752 w815 w864 w930 w979 w1026 w1075 w1122 w1171 w1220 w1260 w1319 w1382 w1388] -> w156
          tunnel: w155 -> [_ w241 _ _ _ _ _ _ _ _ _ _ _ _ _ _ _ _ _ _ _ _ _ _]
          frame "-1", Default {
            n64 = control-ref of="Final Result"() -> (w224:refnum<vi>)
            n65 = control-ref of="Top Result"() -> (w228:refnum<vi>)
            n66 = control-ref of="Bottom Result"() -> (w230:refnum<vi>)
            n67 = control-ref of="Camera Status"() -> (w229:refnum<vi>)
            n68 = control-ref of="Camera Status"() -> (w227:refnum<vi>)
            n69 = control-ref of="Final Result"() -> (w226:refnum<vi>)
            n70 = control-ref of="Final Result"() -> (w220:refnum<vi>)
            n71 = control-ref of="Shaft Status"() -> (w221:refnum<vi>)
            n72 = call "OP10 Indicators.vi"("error in (no error)"=w234, "OUTPUT INDICATOR"=w233, "Boolean in"=w224) -> ("error out"=w223:errorcluster, "OUTPUT INDICATOR"=w232:T11)  [unwired: 7 in]
            n73 = Build Array(w230, w229, w228, w227, w226) -> (w225:refnum<vi>[])
            n74 = Build Array(w221, w220) -> (w219:refnum<vi>[])
            n75 = control-ref of="RH Status"() -> (w216:refnum<vi>)
            n76 = control-ref of="LH Status"() -> (w215:refnum<vi>)
            n77 = control-ref of="Final Result"() -> (w214:refnum<vi>)
            n78 = call "OP20 Indicators.vi"("error in (no error)"=w223, "Array"=w225, "OUTPUT INDICATOR"=w232) -> ("error out"=w222:errorcluster, "OUTPUT INDICATOR"=w231:T11)  [unwired: 7 in]
            n79 = control-ref of="Nut Status"() -> (w210:refnum<vi>)
            n80 = control-ref of="RH Status"() -> (w209:refnum<vi>)
            n81 = control-ref of="LH Status"() -> (w208:refnum<vi>)
            n82 = control-ref of="Camera Status"() -> (w207:refnum<vi>)
            n83 = control-ref of="Final Result"() -> (w206:refnum<vi>)
            n84 = Build Array(w216, w215, w214) -> (w213:refnum<vi>[])
            n85 = call "OP30 Indicators.vi"("error in (no error)"=w222, "Array"=w219, "OUTPUT INDICATOR"=w231) -> ("error out"=w217:errorcluster, "OUTPUT INDICATOR"=w218:T11)  [unwired: 7 in]
            n86 = Build Array(w210, w209, w208, w207, w206) -> (w205:refnum<vi>[])
            n87 = call "OP40 Indicators.vi"("error in (no error)"=w217, "Array"=w213, "OUTPUT INDICATOR"=w218) -> ("error out"=w212:errorcluster, "OUTPUT INDICATOR"=w211:T11)  [unwired: 7 in]
            n88 = control-ref of="Screw 1 Status"() -> (w201:refnum<vi>)
            n89 = control-ref of="Screw 2 Status"() -> (w200:refnum<vi>)
            n90 = control-ref of="Screw 3 Status"() -> (w199:refnum<vi>)
            n91 = control-ref of="Screw 4 Status"() -> (w198:refnum<vi>)
            n92 = control-ref of="Screw 5 Status"() -> (w197:refnum<vi>)
            n93 = control-ref of="Screw 6 Status"() -> (w196:refnum<vi>)
            n94 = control-ref of="Final Result"() -> (w195:refnum<vi>)
            n95 = control-ref of="Final Result"() -> (w192:refnum<vi>)
            n96 = call "OP50 Indicators.vi"("error in (no error)"=w212, "Array"=w205, "OUTPUT INDICATOR"=w211) -> ("error out"=w204:errorcluster, "OUTPUT INDICATOR"=w203:T11)  [unwired: 7 in]
            n97 = Build Array(w201, w200, w199, w198, w197, w196, w195) -> (w202:refnum<vi>[])
            n98 = control-ref of="Loctite Status"() -> (w188:refnum<vi>)
            n99 = control-ref of="Final Result"() -> (w187:refnum<vi>)
            n100 = Build Array(w192) -> (w191:refnum<vi>[])
            n101 = call "OP60 Indicators.vi"("error in (no error)"=w204, "Array"=w202, "OUTPUT INDICATOR"=w203) -> ("error out"=w194:errorcluster, "OUTPUT INDICATOR"=w193:T11)  [unwired: 7 in]
            n102 = call "OP70 Indicators.vi"("error in (no error)"=w194, "Array"=w191, "OUTPUT INDICATOR"=w193) -> ("error out"=w190:errorcluster, "OUTPUT INDICATOR"=w189:T11)  [unwired: 7 in]
            n103 = control-ref of="Seat Status"() -> (w183:refnum<vi>)
            n104 = control-ref of="Final Result"() -> (w182:refnum<vi>)
            n105 = control-ref of="Final Result"() -> (w178:refnum<vi>)
            n106 = Build Array(w188, w187) -> (w186:refnum<vi>[])
            n107 = call "OP80 Indicators.vi"("error in (no error)"=w190, "Array"=w186, "OUTPUT INDICATOR"=w189) -> ("error out"=w184:errorcluster, "OUTPUT INDICATOR"=w185:T11)  [unwired: 7 in]
            n108 = Build Array(w183, w182) -> (w181:refnum<vi>[])
            n109 = Build Array(w178) -> (w177:refnum<vi>[])
            n110 = call "OP90 Indicators.vi"("error in (no error)"=w184, "Array"=w181, "OUTPUT INDICATOR"=w185) -> ("error out"=w180:errorcluster, "OUTPUT INDICATOR"=w179:T11)  [unwired: 7 in]
            n111 = call "OP100 Indicators.vi"("error in (no error)"=w180, "Array"=w177, "OUTPUT INDICATOR"=w179) -> ("error out"=w171:errorcluster, "OUTPUT INDICATOR"=w176:T11)  [unwired: 7 in]
            n112 = call "PADMINI_AUTO_BARCODE_STRING 110.vi"("Enum"=enum16{"Read", "Write"}."Read", "error in (no error)"=w171) -> ("Input 2"=w173:string[])  [unwired: 8 in, 1 out]
            n113 = Index Array(array=w173) -> (element=w174:string)  [unwired: 1 in]
            n114 = Bundle By Name(cluster=w176, "OP - 110.BARCODE"=w174) -> (w175:T11)
          }
          frame "SCAN1" {
            # "STATION OP 10"
            n115 = global read "Global 1.vi" "BARCODE RECIPE"() -> (w248:string)
            n116 = call "PADMINI_AUTO_BARCODE_STRING.vi"("Enum"=enum16{"Read", "Write"}."Read", "error in (no error)"=w257) -> ("error out"=w256:errorcluster, "Input 2"=w244:string[])  [unwired: 8 in]
            n117 = Index Array(array=w244) -> (element=w243:string)  [unwired: 1 in]
            n118 = call <vilib>:"Trim Whitespace.vi"("string"=w243) -> ("trimmed string"=w242:string)  [unwired: 1 in]
            n119 = Match Pattern(string=w242, regular expression=w248) -> (match substring=w251:string)  [unwired: 1 in, 3 out]
            n120 = String Length(string=w248) -> (length=w250:i32)
            n121 = String Length(string=w251) -> (length=w249:i32)
            n122 = Equal?(x=w250, y=w249) -> (x = y?=w255:bool)
            n123 = case shown="False" w254 {
              tunnel: w261 -> [w287 w305]
              tunnel: w256 -> [w286 w303]
              tunnel: w260 -> [w285 _]
              tunnel: [w284 w302] -> w246
              tunnel: [w283 w305] -> w259
              tunnel: w255 -> [_ _]
              tunnel: w242 -> [w282 _]
              tunnel: [w281 TRUE] -> w240
              frame False {
                n124 = Format Into String(format string="where BARCODE='%s'", w282) -> (resulting string=w278:string)  [unwired: 2 in, 1 out]
                n125 = call <vilib>:"DB Tools Select Data.vi"("condition"=w278, "error in (no error)"=w286, "columns"=string[] ["BARCODE", "OP10_FINAL_RST"], "table"=w285, "connection reference"=w287) -> ("error out"=w277:errorcluster, "data"=w276:variant[][], "connection reference out"=w283:T13)  [unwired: 1 in]
                n126 = call "PADMINI_varient_to_data.vi"("error in (no error)"=w277, "data"=w276) -> ("error out"=w274:errorcluster, "Array"=w270:string[][])  [unwired: 8 in]
                n127 = Index Array(array=w270, index (row)=0) -> (element=→"SCAN OP10":string[])  [unwired: 1 in]
                n128 = Index Array(array=w270, index (row)=0, index (col)=1 ("index (row)")) -> (element=w271:string)
                n129 = Empty Array?(array=w270) -> (empty?=w275:bool)
                n130 = case shown="False" w275 {
                  tunnel: w274 -> [w297 w299]
                  tunnel: [w296 w299] -> w284
                  tunnel: [FALSE TRUE] -> w281
                  tunnel: w271 -> [w291 _]
                  frame False {
                    w290 = "OK"  # y
                    w293 = i32[] [1, 0]  # I/P
                    w292 = i32[] [0, 1]  # I/P
                    # "OP10 CURRENT STATION OK-NG\nPART REPEAT"
                    n131 = Equal?(x=w291, y=w290) -> (x = y?=w289:bool)
                    n132 = Select(t=w293, s=w289, f=w292) -> (s? t:f=w288:i32[])
                    "OP10 STATUS" <- w288
                    n133 = call "PADMINI_AUTO_BARCODE_STATUS.vi"("Enum"=enum16{"Read", "Write"}."Write", "error in (no error)"=w297, "I/P"=w288) -> ("error out"=w296:errorcluster)  [unwired: 7 in, 1 out]
                  }
                  frame True {
                    # "OP10 NEW part"
                  }
                }
              }
              frame True {
                w301 = i32[] [0, 1]  # I/P
                n134 = call "PADMINI_AUTO_BARCODE_STATUS.vi"("Enum"=enum16{"Read", "Write"}."Write", "error in (no error)"=w303, "I/P"=w301) -> ("error out"=w302:errorcluster)  [unwired: 7 in, 1 out]
              }
            }
            n135 = flat-sequence {
              tunnel: [w267] -> w245
              tunnel: w246 -> [w267]
              frame #0 {
                # "UPDATE op 10 sCAN sTATUS"
                n136 = global write "DATA LOG.vi" "OP 10 Outputs"(TRUE) -> ()
              }
            }
            n137 = call <vilib>:"Clear Errors.vi"("error in (no error)"=w245) -> ("error out"=w239:errorcluster)  [unwired: 5 in, 1 out]
            n138 = case shown="True" w240 {
              tunnel: w241 -> [_ w265]
              tunnel: w239 -> [_ w263]
              frame False {
              }
              frame True {
                w264 = cluster{"CASE 2":T12} {"CASE 2"=enum."DATALOG1"}  # element
                n139 = Enqueue Element(queue=w265, element=w264, error in (no error)=w263) -> ()  [unwired: 1 in, 3 out]
              }
            }
          }
          frame "DATALOG1" {
            w320 = T14 2 items=["no dialog", "OK message", "continue or stop message", "OK message + warnings", "continue/stop + warnings"] ("type of dialog (OK msg:1)")
            # "cycle result status\nwhether it was ok or nok\nor abortted in between"
            # "Printed QR Code data string"
            # "datalog of OP 10"
            n140 = call "PADMINI_AUTO_BARCODE_STRING.vi"("Enum"=enum16{"Read", "Write"}."Read", "error in (no error)"=w306) -> ("Input 2"=w313:string[])  [unwired: 8 in, 1 out]
            n141 = call "PADMINI_AUTO_CYCLE VALUE 10.vi"("Enum"=enum16{"Read", "Write"}."Read", "error in (no error)"=w306) -> ("error out"=w309:errorcluster, "Input 2"=w308:sgl[])  [unwired: 8 in]
            n142 = Index Array(array=w308) -> (element=w307:sgl)  [unwired: 1 in]
            n143 = Index Array(array=w313) -> (element #1=w312:string, element #2=w311:string)  [unwired: 2 in]
            n144 = Number To Fractional String(number=w307, precision (6)=i16 2) -> (F-format string=w314:string)  [unwired: 2 in]
            n145 = call <vilib>:"Trim Whitespace.vi"("string"=w312) -> ("trimmed string"=w323:string)  [unwired: 1 in]
            n146 = case shown="False" w328 {
              tunnel: w329 -> [w353 w388]
              tunnel: w309 -> [w355 w387]
              tunnel: [w361 w386] -> w326
              tunnel: [w360 w385] -> w321
              tunnel: w327 -> [w350 _]
              tunnel: w323 -> [w347 _]
              tunnel: w311 -> [w357 w378]
              tunnel: w314 -> [w341 w377]
              frame False {
                w349 = string[] ["BARCODE", "SHIFT", "OP10_DATE", "OP10_LEAK_RATE", "OP10_FINAL_RST"]
                # "ST1 RESULT"
                # "DO TRACEBILITY"
                n147 = local read "SHIFT"() -> (w359:string)
                n148 = Format Into String(format string="Where BARCODE='%s' ", w347) -> (resulting string=w342:string)  [unwired: 2 in, 1 out]
                n149 = call <vilib>:"DB Tools Select Data.vi"("condition"=w342, "error in (no error)"=w355, "columns"=w349, "table"=w350, "connection reference"=w353) -> ("error out"=w351:errorcluster, "data"=w354:variant[][], "connection reference out"=w352:T13)  [unwired: 1 in]
                n150 = call "PADMINI_SHIFT_DATE.vi"("SHIFT"=w359) -> ("date/time string"=w358:string)  [unwired: 10 in]
                n151 = Variant To Data(error in=w351, type=string[][] [], Variant=w354) -> (data=w345:string[][], error out=w343:errorcluster)
                n152 = Bundle("trimmed string"=w347, "SHIFT"=w359, "date/time string"=w358, w341, "Input 2"=w357) -> (w356:T15)  [unwired: 1 in]
                n153 = Empty Array?(array=w345) -> (empty?=w344:bool)
                n154 = case shown="False" w344 {
                  tunnel: w352 -> [w366 w376]
                  tunnel: w343 -> [w365 w375]
                  tunnel: [w369 w374] -> w361
                  tunnel: [w368 w373] -> w360
                  tunnel: w349 -> [w363 w372]
                  tunnel: w350 -> [w364 w371]
                  tunnel: w356 -> [w367 w370]
                  tunnel: w342 -> [w362 _]
                  frame False {
                    n155 = call <vilib>:"DB Tools Update Data.vi"("condition"=w362, "data"=w367, "error in (no error)"=w365, "columns"=w363, "table"=w364, "connection reference"=w366) -> ("error out"=w368:errorcluster, "connection reference out"=w369:T13)  [unwired: 4 in]
                  }
                  frame True {
                    n156 = call <vilib>:"DB Tools Insert Data.vi"("data"=w370, "error in (no error)"=w375, "columns"=w372, "table"=w371, "connection reference"=w376) -> ("error out"=w373:errorcluster, "connection reference out"=w374:T13)  [unwired: 5 in]
                  }
                }
              }
              frame True {
                # "Trac BYPASS"
                n157 = local read "SHIFT"() -> (w383:string)
                n158 = call "PADMINI_SHIFT_DATE.vi"("SHIFT"=w383) -> ("date/time string"=w382:string)  [unwired: 10 in]
                n159 = Bundle("SHIFT"=w383, "date/time string"=w382, "Input 2"=w378, w377) -> (w381:T16)  [unwired: 1 in]
                n160 = To Variant(anything=w381) -> (Variant=w380:variant)
                n161 = call <vilib>:"DB Tools Insert Data.vi"("data"=w380, "error in (no error)"=w387, "columns"=string[] ["DATE", "SHIFT", "OP10_LEAK_RAT", "OP10_FINAL_RST"], "table"="ST1_REPORT", "connection reference"=w388) -> ("error out"=w385:errorcluster, "connection reference out"=w386:T13)  [unwired: 5 in]
              }
            }
            n162 = call <vilib>:"Simple Error Handler.vi"("type of dialog (OK msg:1)"=w320, "error in (no error)"=w321) -> ("error out"=w319:errorcluster)  [unwired: 3 in, 4 out]
            n163 = call <vilib>:"Clear Errors.vi"("error in (no error)"=w319) -> ("error out"=w317:errorcluster)  [unwired: 5 in, 1 out]
            n164 = disable-structure shown="Enabled" {
              disable-tunnel: [w339 w340] -> w325
              disable-tunnel: w317 -> [w338 w340]
              frame Disabled {
                w333 = refnum<vi> refnum  # Boolean
                n165 = property on="OP - 10" class="Clust"(error in=w338) -> (error out=w332:errorcluster, "Controls[]"=w336:refnum<vi>[])  [unwired: 1 in, 1 out]
                n166 = Index Array(array=w336, index=2) -> (element=w334:refnum<vi>)
                n167 = To More Specific Class(target class=w333, reference=w334, error in=w332) -> (specific class reference=w337:refnum<vi>, error out=w331:errorcluster)
                n168 = call "PADMINI_BOOL_COLOR_CHANGE.vi"("error in (no error)"=w331, "Boolean in"=w337) -> ("error out"=w339:errorcluster)  [unwired: 9 in]
              }
              frame Enabled {
              }
            }
          }
          frame "SCAN2" {
            # "Barcode Status\n0-Ideal, 1-Ok, 2-Nok, 3-Prev Station Not Done,\n4-Prev Station Nok,\n5- Already Done"
            # "STATION OP 20"
            n169 = case shown="False" w395 {
              tunnel: w399 -> [w424 w430]
              tunnel: w398 -> [w417 w428]
              tunnel: w397 -> [w405 _]
              tunnel: [w419 w427] -> w394
              tunnel: [w418 w430] -> w396
              tunnel: [w406 "" ("trimmed string")] -> _
              frame False {
                # "ST2 RESULT"
                # "ST1 RESULT"
                # "2 FOR EMPTY BARCODE READ OR MISMATCH"
                n170 = call "PADMINI_AUTO_BARCODE_STRING2.vi"("Enum"=enum16{"Read", "Write"}."Read", "error in (no error)"=w417) -> ("error out"=w416:errorcluster, "Input 2"=w408:string[])  [unwired: 8 in]
                n171 = global read "Global 1.vi" "BARCODE RECIPE"() -> (w409:string)
                n172 = Index Array(array=w408) -> (element=w407:string)  [unwired: 1 in]
                n173 = call <vilib>:"Trim Whitespace.vi"("string"=w407) -> ("trimmed string"=w406:string)  [unwired: 1 in]
                n174 = Match Pattern(string=w406, regular expression=w409) -> (match substring=w410:string)  [unwired: 1 in, 3 out]
                n175 = String Length(string=w409) -> (length=w412:i32)
                n176 = String Length(string=w410) -> (length=w411:i32)
                n177 = Format Into String(format string="WHERE BARCODE  ='%s'", w406) -> (resulting string=w413:string)  [unwired: 2 in, 1 out]
                n178 = Equal?(x=w412, y=w411) -> ()  [unwired: 1 out]
                n179 = call <vilib>:"DB Tools Select Data.vi"("condition"=w413, "error in (no error)"=w416, "columns"=string[] ["BARCODE", "OP10_FINAL_RST", "OP20_FINAL_RST"], "table"=w405, "connection reference"=w424) -> ("error out"=w422:errorcluster, "data"=w421:variant[][], "connection reference out"=w418:T13)  [unwired: 1 in]
                n180 = call "PADMINI_varient_to_data.vi"("error in (no error)"=w422, "data"=w421) -> ("error out"=w420:errorcluster, "Array"=w402:string[][])  [unwired: 8 in]
                n181 = Index Array(array=w402, index (row)=0 ("disabled index (col)")) -> (element=→"SCAN OP20":string[])  [unwired: 1 in]
                n182 = call "RESPONSE_LOGIC.vi"("Array"=w402) -> ("Not Found"=w400:i32[])  [unwired: 10 in]
                "OP20 STATUS" <- w400
                n183 = call "PADMINI_AUTO_BARCODE_STATUS 20.vi"("Enum"=enum16{"Read", "Write"}."Write", "error in (no error)"=w420, "I/P"=w400) -> ("error out"=w419:errorcluster)  [unwired: 7 in, 1 out]
              }
              frame True {
                w425 = i32[] [0, 0, 0, 0, 0]  # I/P
                n184 = call "PADMINI_AUTO_BARCODE_STATUS 20.vi"("Enum"=enum16{"Read", "Write"}."Write", "error in (no error)"=w428, "I/P"=w425) -> ("error out"=w427:errorcluster)  [unwired: 7 in, 1 out]
              }
            }
            n185 = flat-sequence {
              tunnel: [w432] -> w393
              tunnel: w394 -> [w432]
              frame #0 {
                # "UPDATE op 20 SCAN sTATUS"
                n186 = global write "DATA LOG.vi" "OP 20 Outputs"(TRUE) -> ()
              }
            }
          }
          frame "DATALOG2" {
            w446 = T14 2 items=["no dialog", "OK message", "continue or stop message", "OK message + warnings", "continue/stop + warnings"] ("type of dialog (OK msg:1)")
            # "Printed QR Code data string"
            # "datalog of OP 20"
            n187 = call "PADMINI_AUTO_BARCODE_STRING2.vi"("Enum"=enum16{"Read", "Write"}."Read", "error in (no error)"=w439) -> ("error out"=w441:errorcluster, "Input 2"=w435:string[])  [unwired: 8 in]
            n188 = call "PADMINI_AUTO_CYCLE VALUE 20.vi"("Enum"=enum16{"Read", "Write"}."Read", "error in (no error)"=w439) -> ("Input 2"=w437:sgl[])  [unwired: 8 in, 1 out]
            n189 = Number To Fractional String(number=w437, precision (6)=i16 2) -> (F-format string=w436:string[])  [unwired: 2 in]
            n190 = case shown="False" w451 {
              tunnel: w452 -> [w476 w502]
              tunnel: w441 -> [w477 w501]
              tunnel: [w480 w500] -> w449
              tunnel: [w479 w499] -> w447
              tunnel: w450 -> [w475 _]
              tunnel: w436 -> [w472 w484]
              tunnel: w435 -> [w466 w485]
              frame False {
                # "ST2 RESULT"
                # "DO TRACEBILITY"
                n191 = Index Array(array=w466) -> (element #1=w467:string, element #2=w461:string, element #3=w460:string, element #4=w459:string, element #5=w458:string, element #6=w457:string, element #7=w456:string)  [unwired: 7 in]
                n192 = local read "SHIFT"() -> (w478:string)
                n193 = Index Array(array=w472) -> (element #1=w471:string, element #2=w470:string, element #3=w463:string, element #4=w462:string)  [unwired: 4 in]
                n194 = call <vilib>:"Trim Whitespace.vi"("string"=w467) -> ("trimmed string"=w468:string)  [unwired: 1 in]
                n195 = call "PADMINI_SHIFT_DATE.vi"("SHIFT"=w478) -> ("date/time string"=w465:string)  [unwired: 10 in]
                n196 = Format Into String(format string="Where BARCODE='%s' ", w468) -> (resulting string=w473:string)  [unwired: 2 in, 1 out]
                n197 = Bundle("date/time string"=w465, "Input 2"=w471, "Input 2"=w470, "Input 2"=w463, "Input 2"=w462, "Input 2"=w461, "Input 2"=w460, "Input 2"=w459, "Input 2"=w458, "Input 2"=w457, "Input 2"=w456) -> (w469:T17)  [unwired: 1 in]
                n198 = call <vilib>:"DB Tools Update Data.vi"("condition"=w473, "data"=w469, "error in (no error)"=w477, "columns"=string[] ["OP20_DATE", "OP20_LOWER_BEARING_DIS", "OP20_LOWER_BEARING_LOAD", "OP20_UPPER_BEARING_DIS", "OP20_UPPER_BEARING_LOAD", "OP20_LOWER_BEARING_RST", "OP20_BOTTOM_CAMERA_STATUS", "OP20_UPPER_SIM_STATUS", "OP20_UPPER_BERAING_RST", "OP20_UPPER_CAMERA_STATUS", "OP20_FINAL_RST"], "table"=w475, "connection reference"=w476) -> ("error out"=w479:errorcluster, "connection reference out"=w480:T13)  [unwired: 4 in]
              }
              frame True {
                n199 = local read "SHIFT"() -> (w482:string)
                n200 = Index Array(array=w485) -> (element #2=w491:string, element #3=w490:string, element #4=w489:string, element #5=w488:string, element #6=w487:string, element #7=w481:string)  [unwired: 7 in, 1 out]
                n201 = call "PADMINI_SHIFT_DATE.vi"("SHIFT"=w482) -> ("date/time string"=w483:string)  [unwired: 10 in]
                n202 = Index Array(array=w484) -> (element #1=w495:string, element #2=w494:string, element #3=w493:string, element #4=w492:string)  [unwired: 4 in]
                n203 = Bundle("date/time string"=w483, "SHIFT"=w482, "Input 2"=w495, "Input 2"=w494, "Input 2"=w491, "Input 2"=w490, "Input 2"=w493, "Input 2"=w492, "Input 2"=w489, "Input 2"=w488, "Input 2"=w487, "Input 2"=w481) -> (w486:T18)  [unwired: 1 in]
                n204 = To Variant(anything=w486) -> (Variant=w497:variant)
                n205 = call <vilib>:"DB Tools Insert Data.vi"("data"=w497, "error in (no error)"=w501, "columns"=string[] ["DATE", "SHIFT", "ST2_LOWER_BEARING_DIS", "ST2_LOWER_BEARING_LOAD", "ST2_BOTTOM_CAMERA_STATUS", "ST2_LOWER_BEARING_RST", "ST2_UPPER_BEARING_DIS", "ST2_UPPER_BEARING_LOAD", "ST2_UPPER_SIM_STATUS", "ST2_UPPER_CAMERA_STATUS", "ST2_UPPER_BERAING_RST", "ST2_FINAL_RST"], "table"="ST2_REPORT", "connection reference"=w502) -> ("error out"=w499:errorcluster, "connection reference out"=w500:T13)  [unwired: 5 in]
              }
            }
            n206 = call <vilib>:"Simple Error Handler.vi"("type of dialog (OK msg:1)"=w446, "error in (no error)"=w447) -> ("error out"=w445:errorcluster)  [unwired: 3 in, 4 out]
            n207 = call <vilib>:"Clear Errors.vi"("error in (no error)"=w445) -> ("error out"=w443:errorcluster)  [unwired: 5 in, 1 out]
            n208 = flat-sequence {
              tunnel: [w455] -> w434
              tunnel: w443 -> [w455]
              frame #0 {
                # "UPDATE op 20 save"
                n209 = global write "DATA LOG.vi" "OP 20 reset"(TRUE) -> ()
              }
            }
          }
          frame "SCAN3" {
            # "STATION OP 30"
            n210 = case shown="False" w509 {
              tunnel: w513 -> [w539 w545]
              tunnel: w512 -> [w532 w543]
              tunnel: w511 -> [w519 _]
              tunnel: [w534 w542] -> w508
              tunnel: [w533 w545] -> w510
              tunnel: [w520 "" ("trimmed string")] -> _
              frame False {
                n211 = call "PADMINI_AUTO_BARCODE_STRING 30.vi"("Enum"=enum16{"Read", "Write"}."Read", "error in (no error)"=w532) -> ("error out"=w531:errorcluster, "Input 2"=w522:string[])  [unwired: 8 in]
                n212 = global read "Global 1.vi" "BARCODE RECIPE"() -> (w523:string)
                n213 = Index Array(array=w522) -> (element=w521:string)  [unwired: 1 in]
                n214 = call <vilib>:"Trim Whitespace.vi"("string"=w521) -> ("trimmed string"=w520:string)  [unwired: 1 in]
                n215 = Match Pattern(string=w520, regular expression=w523) -> (match substring=w524:string)  [unwired: 1 in, 3 out]
                n216 = String Length(string=w523) -> (length=w526:i32)
                n217 = String Length(string=w524) -> (length=w525:i32)
                n218 = Equal?(x=w520, y="") -> ()  [unwired: 1 out]
                n219 = Format Into String(format string="WHERE BARCODE  ='%s'", w520) -> (resulting string=w528:string)  [unwired: 2 in, 1 out]
                n220 = Equal?(x=w526, y=w525) -> ()  [unwired: 1 out]
                n221 = call <vilib>:"DB Tools Select Data.vi"("condition"=w528, "error in (no error)"=w531, "columns"=string[] ["BARCODE", "OP20_FINAL_RST", "OP30_FINAL_RST"], "table"=w519, "connection reference"=w539) -> ("error out"=w537:errorcluster, "data"=w536:variant[][], "connection reference out"=w533:T13)  [unwired: 1 in]
                n222 = call "PADMINI_varient_to_data.vi"("error in (no error)"=w537, "data"=w536) -> ("error out"=w535:errorcluster, "Array"=w516:string[][])  [unwired: 8 in]
                n223 = Index Array(array=w516, index (row)=0 ("disabled index (col)")) -> (element=→"SCAN OP30":string[])  [unwired: 1 in]
                n224 = call "RESPONSE_LOGIC.vi"("Array"=w516) -> ("Not Found"=w514:i32[])  [unwired: 10 in]
                "OP30 STATUS" <- w514
                n225 = call "PADMINI_AUTO_BARCODE_STATUS 30.vi"("Enum"=enum16{"Read", "Write"}."Write", "error in (no error)"=w535, "I/P"=w514) -> ("error out"=w534:errorcluster)  [unwired: 7 in, 1 out]
              }
              frame True {
                w540 = i32[] [0, 0, 0, 0, 0]  # I/P
                n226 = call "PADMINI_AUTO_BARCODE_STATUS 30.vi"("Enum"=enum16{"Read", "Write"}."Write", "error in (no error)"=w543, "I/P"=w540) -> ("error out"=w542:errorcluster)  [unwired: 7 in, 1 out]
              }
            }
            n227 = flat-sequence {
              tunnel: [w547] -> w507
              tunnel: w508 -> [w547]
              frame #0 {
                # "UPDATE op 30 SCAN sTATUS"
                n228 = global write "DATA LOG.vi" "OP 30 Outputs"(TRUE) -> ()
              }
            }
          }
          frame "DATALOG3" {
            w561 = T14 2 items=["no dialog", "OK message", "continue or stop message", "OK message + warnings", "continue/stop + warnings"] ("type of dialog (OK msg:1)")
            # "Printed QR Code data string"
            # "datalog of OP 30"
            n229 = call "PADMINI_AUTO_BARCODE_STRING 30.vi"("Enum"=enum16{"Read", "Write"}."Read", "error in (no error)"=w553) -> ("error out"=w555:errorcluster, "Input 2"=w549:string[])  [unwired: 8 in]
            n230 = call "PADMINI_AUTO_CYCLE VALUE 30.vi"("Enum"=enum16{"Read", "Write"}."Read", "error in (no error)"=w553) -> ("Input 2"=w551:sgl[])  [unwired: 8 in, 1 out]
            n231 = Number To Fractional String(number=w551, precision (6)=i16 2) -> (F-format string=w550:string[])  [unwired: 2 in]
            n232 = case shown="False" w566 {
              tunnel: w567 -> [w585 w605]
              tunnel: w555 -> [w586 w604]
              tunnel: [w589 w603] -> w564
              tunnel: [w588 w602] -> w562
              tunnel: w565 -> [w584 _]
              tunnel: w550 -> [w580 w590]
              tunnel: w549 -> [w574 w591]
              frame False {
                # "DO TRACEBILITY"
                n233 = Index Array(array=w574) -> (element #1=w575:string, element #2=w573:string, element #3=w572:string)  [unwired: 3 in]
                n234 = local read "SHIFT"() -> (w587:string)
                n235 = Index Array(array=w580) -> (element #1=w579:string, element #2=w578:string)  [unwired: 2 in]
                n236 = call <vilib>:"Trim Whitespace.vi"("string"=w575) -> ("trimmed string"=w576:string)  [unwired: 1 in]
                n237 = call "PADMINI_SHIFT_DATE.vi"("SHIFT"=w587) -> ("date/time string"=w571:string)  [unwired: 10 in]
                n238 = Format Into String(format string="Where BARCODE='%s' ", w576) -> (resulting string=w582:string)  [unwired: 2 in, 1 out]
                n239 = Bundle("date/time string"=w571, "Input 2"=w579, "Input 2"=w578, "Input 2"=w573, "Input 2"=w572) -> (w577:T19)  [unwired: 1 in]
                n240 = call <vilib>:"DB Tools Update Data.vi"("condition"=w582, "data"=w577, "error in (no error)"=w586, "columns"=string[] ["OP30_DATE", "OP30_DISPLACEMENT", "OP30_SHAFT_PRESS_LOAD", "OP30_SHAFT_STATUS", "OP30_FINAL_RST"], "table"=w584, "connection reference"=w585) -> ("error out"=w588:errorcluster, "connection reference out"=w589:T13)  [unwired: 4 in]
              }
              frame True {
                # "TRAC BYPASS"
                n241 = local read "SHIFT"() -> (w592:string)
                n242 = call "PADMINI_SHIFT_DATE.vi"("SHIFT"=w592) -> ("date/time string"=w593:string)  [unwired: 10 in]
                n243 = Index Array(array=w591) -> (element #2=w597:string, element #3=w596:string)  [unwired: 3 in, 1 out]
                n244 = Index Array(array=w590) -> (element #1=w599:string, element #2=w598:string)  [unwired: 2 in]
                n245 = Bundle("date/time string"=w593, "SHIFT"=w592, "Input 2"=w599, "Input 2"=w598, "Input 2"=w597, "Input 2"=w596) -> (w594:T20)  [unwired: 1 in]
                n246 = To Variant(anything=w594) -> (Variant=w595:variant)
                n247 = call <vilib>:"DB Tools Insert Data.vi"("data"=w595, "error in (no error)"=w604, "columns"=string[] ["DATE", "SHIFT", "ST3_DISPLACEMENT", "ST3_LOAD", "ST3_MIDDLE_GEAR_SHAFT_STATUS", "ST3_FINAL_RST"], "table"="ST3_REPORT", "connection reference"=w605) -> ("error out"=w602:errorcluster, "connection reference out"=w603:T13)  [unwired: 5 in]
              }
            }
            n248 = call <vilib>:"Simple Error Handler.vi"("type of dialog (OK msg:1)"=w561, "error in (no error)"=w562) -> ("error out"=w560:errorcluster)  [unwired: 3 in, 4 out]
            n249 = call <vilib>:"Clear Errors.vi"("error in (no error)"=w560) -> ("error out"=w558:errorcluster)  [unwired: 5 in, 1 out]
            n250 = flat-sequence {
              tunnel: [w570] -> w548
              tunnel: w558 -> [w570]
              frame #0 {
                # "UPDATE op 20 save"
                n251 = global write "DATA LOG.vi" "OP 30 reset"(TRUE) -> ()
              }
            }
          }
          frame "SCAN4" {
            # "STATION OP 40"
            n252 = case shown="False" w612 {
              tunnel: w616 -> [w637 w643]
              tunnel: w615 -> [w630 w642]
              tunnel: w614 -> [w622 _]
              tunnel: [w632 w641] -> w611
              tunnel: [w631 w643] -> w613
              tunnel: [w623 "" ("trimmed string")] -> _
              frame False {
                n253 = call "PADMINI_AUTO_BARCODE_STRING 40.vi"("Enum"=enum16{"Read", "Write"}."Read", "error in (no error)"=w630) -> ("error out"=w629:errorcluster, "Input 2"=w625:string[])  [unwired: 8 in]
                n254 = Index Array(array=w625) -> (element=w624:string)  [unwired: 1 in]
                n255 = call <vilib>:"Trim Whitespace.vi"("string"=w624) -> ("trimmed string"=w623:string)  [unwired: 1 in]
                n256 = Format Into String(format string="WHERE BARCODE  ='%s'", w623) -> (resulting string=w626:string)  [unwired: 2 in, 1 out]
                n257 = call <vilib>:"DB Tools Select Data.vi"("condition"=w626, "error in (no error)"=w629, "columns"=string[] ["BARCODE", "OP30_FINAL_RST", "OP40_FINAL_RST"], "table"=w622, "connection reference"=w637) -> ("error out"=w635:errorcluster, "data"=w634:variant[][], "connection reference out"=w631:T13)  [unwired: 1 in]
                n258 = call "PADMINI_varient_to_data.vi"("error in (no error)"=w635, "data"=w634) -> ("error out"=w633:errorcluster, "Array"=w619:string[][])  [unwired: 8 in]
                n259 = call "RESPONSE_LOGIC.vi"("Array"=w619) -> ("Not Found"=w617:i32[])  [unwired: 10 in]
                "OP40 STATUS" <- w617
                n260 = Index Array(array=w619, index (row)=0 ("disabled index (col)")) -> (element=→"SCAN OP40":string[])  [unwired: 1 in]
                n261 = call "PADMINI_AUTO_BARCODE_STATUS 40.vi"("Enum"=enum16{"Read", "Write"}."Write", "error in (no error)"=w633, "I/P"=w617) -> ("error out"=w632:errorcluster)  [unwired: 7 in, 1 out]
              }
              frame True {
                w638 = i32[] [0, 0, 0, 0, 0]  # I/P
                n262 = call "PADMINI_AUTO_BARCODE_STATUS 40.vi"("Enum"=enum16{"Read", "Write"}."Write", "error in (no error)"=w642, "I/P"=w638) -> ("error out"=w641:errorcluster)  [unwired: 7 in, 1 out]
              }
            }
            n263 = flat-sequence {
              tunnel: [w645] -> w610
              tunnel: w611 -> [w645]
              frame #0 {
                # "UPDATE op 40 SCAN sTATUS"
                n264 = global write "DATA LOG.vi" "OP 40 Outputs"(TRUE) -> ()
              }
            }
          }
          frame "DATALOG4" {
            w659 = T14 2 items=["no dialog", "OK message", "continue or stop message", "OK message + warnings", "continue/stop + warnings"] ("type of dialog (OK msg:1)")
            # "datalog of OP 40"
            n265 = call "PADMINI_AUTO_BARCODE_STRING 40.vi"("Enum"=enum16{"Read", "Write"}."Read", "error in (no error)"=w651) -> ("error out"=w653:errorcluster, "Input 2"=w647:string[])  [unwired: 8 in]
            n266 = call "PADMINI_AUTO_CYCLE VALUE 40.vi"("Enum"=enum16{"Read", "Write"}."Read", "error in (no error)"=w651) -> ("Input 2"=w649:sgl[])  [unwired: 8 in, 1 out]
            n267 = Number To Fractional String(number=w649, precision (6)=i16 2) -> (F-format string=w648:string[])  [unwired: 2 in]
            n268 = case shown="False" w664 {
              tunnel: w665 -> [w687 w711]
              tunnel: w653 -> [w688 w710]
              tunnel: [w691 w709] -> w662
              tunnel: [w690 w708] -> w660
              tunnel: w663 -> [w686 _]
              tunnel: w648 -> [w682 w693]
              tunnel: w647 -> [w677 w692]
              frame False {
                # "DO TRACEBILITY"
                n269 = Index Array(array=w677) -> (element #1=w678:string, element #2=w673:string, element #3=w672:string, element #4=w671:string, element #5=w670:string)  [unwired: 5 in]
                n270 = local read "SHIFT"() -> (w689:string)
                n271 = Index Array(array=w682) -> (element #1=w681:string, element #2=w676:string, element #3=w675:string, element #4=w674:string)  [unwired: 4 in]
                n272 = call <vilib>:"Trim Whitespace.vi"("string"=w678) -> ("trimmed string"=w679:string)  [unwired: 1 in]
                n273 = call "PADMINI_SHIFT_DATE.vi"("SHIFT"=w689) -> ("date/time string"=w669:string)  [unwired: 10 in]
                n274 = Format Into String(format string="Where BARCODE='%s' ", w679) -> (resulting string=w684:string)  [unwired: 2 in, 1 out]
                n275 = Bundle("date/time string"=w669, "Input 2"=w681, "Input 2"=w673, "Input 2"=w676, "Input 2"=w672, "Input 2"=w675, "Input 2"=w674, "Input 2"=w670, "Input 2"=w671) -> (w680:T21)  [unwired: 1 in]
                n276 = call <vilib>:"DB Tools Update Data.vi"("condition"=w684, "data"=w680, "error in (no error)"=w688, "columns"=string[] ["OP40_DATE", "OP40_RH_SCREW", "OP40_RH_STATUS", "OP40_LH_SCREW", "OP40_LH_STATUS", "OP40_DISPLACEMENT", "OP40_STACK_LOAD", "OP40_TOP_BEARING_CAMERA_STAUS", "OP40_FINAL_RST"], "table"=w686, "connection reference"=w687) -> ("error out"=w690:errorcluster, "connection reference out"=w691:T13)  [unwired: 4 in]
              }
              frame True {
                # "TRAC BYPASS"
                n277 = local read "SHIFT"() -> (w694:string)
                n278 = Index Array(array=w692) -> (element #2=w702:string, element #3=w701:string, element #4=w700:string, element #5=w699:string)  [unwired: 5 in, 1 out]
                n279 = call "PADMINI_SHIFT_DATE.vi"("SHIFT"=w694) -> ("date/time string"=w695:string)  [unwired: 10 in]
                n280 = Index Array(array=w693) -> (element #1=w696:string, element #2=w705:string, element #3=w704:string, element #4=w703:string)  [unwired: 4 in]
                n281 = Bundle("date/time string"=w695, "SHIFT"=w694, "Input 2"=w696, "Input 2"=w702, "Input 2"=w705, "Input 2"=w701, "Input 2"=w704, "Input 2"=w703, "Input 2"=w699, "Input 2"=w700) -> (w698:T22)  [unwired: 1 in]
                n282 = To Variant(anything=w698) -> (Variant=w697:variant)
                n283 = call <vilib>:"DB Tools Insert Data.vi"("data"=w697, "error in (no error)"=w710, "columns"=string[] ["DATE", "SHIFT", "ST4_SCREW1_DATA", "ST4_SCREW1_STATUS", "ST4_SCREW2_DATA", "ST4_SCREW2_STATUS", "ST4_DISPLACEMENT", "ST4_LOAD", "ST4_TOP_BEARING_CAMERA_STAUS", "ST4_FINAL_RST"], "table"="ST4_REPORT", "connection reference"=w711) -> ("error out"=w708:errorcluster, "connection reference out"=w709:T13)  [unwired: 5 in]
              }
            }
            n284 = call <vilib>:"Simple Error Handler.vi"("type of dialog (OK msg:1)"=w659, "error in (no error)"=w660) -> ("error out"=w658:errorcluster)  [unwired: 3 in, 4 out]
            n285 = call <vilib>:"Clear Errors.vi"("error in (no error)"=w658) -> ("error out"=w656:errorcluster)  [unwired: 5 in, 1 out]
            n286 = flat-sequence {
              tunnel: [w668] -> w646
              tunnel: w656 -> [w668]
              frame #0 {
                # "UPDATE op 20 save"
                n287 = global write "DATA LOG.vi" "OP 40 reset"(TRUE) -> ()
              }
            }
          }
          frame "SCAN5" {
            # "STATION OP 50"
            n288 = case shown="False" w718 {
              tunnel: w722 -> [w743 w749]
              tunnel: w721 -> [w736 w748]
              tunnel: w720 -> [w728 _]
              tunnel: [w738 w747] -> w717
              tunnel: [w737 w749] -> w719
              tunnel: [w729 "" ("trimmed string")] -> _
              frame False {
                n289 = call "PADMINI_AUTO_BARCODE_STRING 50.vi"("Enum"=enum16{"Read", "Write"}."Read", "error in (no error)"=w736) -> ("error out"=w735:errorcluster, "Input 2"=w731:string[])  [unwired: 8 in]
                n290 = Index Array(array=w731) -> (element=w730:string)  [unwired: 1 in]
                n291 = call <vilib>:"Trim Whitespace.vi"("string"=w730) -> ("trimmed string"=w729:string)  [unwired: 1 in]
                n292 = Format Into String(format string="WHERE BARCODE  ='%s'", w729) -> (resulting string=w732:string)  [unwired: 2 in, 1 out]
                n293 = call <vilib>:"DB Tools Select Data.vi"("condition"=w732, "error in (no error)"=w735, "columns"=string[] ["BARCODE", "OP40_FINAL_RST", "OP50_FINAL_RST"], "table"=w728, "connection reference"=w743) -> ("error out"=w741:errorcluster, "data"=w740:variant[][], "connection reference out"=w737:T13)  [unwired: 1 in]
                n294 = call "PADMINI_varient_to_data.vi"("error in (no error)"=w741, "data"=w740) -> ("error out"=w739:errorcluster, "Array"=w725:string[][])  [unwired: 8 in]
                n295 = Index Array(array=w725, index (row)=0 ("disabled index (col)")) -> (element=→"SCAN OP50":string[])  [unwired: 1 in]
                n296 = call "RESPONSE_LOGIC.vi"("Array"=w725) -> ("Not Found"=w724:i32[])  [unwired: 10 in]
                "OP50 STATUS" <- w724
                n297 = call "PADMINI_AUTO_BARCODE_STATUS 50.vi"("Enum"=enum16{"Read", "Write"}."Write", "error in (no error)"=w739, "I/P"=w724) -> ("error out"=w738:errorcluster)  [unwired: 7 in, 1 out]
              }
              frame True {
                w744 = i32[] [0, 0, 0, 0, 0]  # I/P
                n298 = call "PADMINI_AUTO_BARCODE_STATUS 50.vi"("Enum"=enum16{"Read", "Write"}."Write", "error in (no error)"=w748, "I/P"=w744) -> ("error out"=w747:errorcluster)  [unwired: 7 in, 1 out]
              }
            }
            n299 = flat-sequence {
              tunnel: [w751] -> w716
              tunnel: w717 -> [w751]
              frame #0 {
                # "UPDATE op 50 SCAN sTATUS"
                n300 = global write "DATA LOG.vi" "OP 50 Outputs"(TRUE) -> ()
              }
            }
          }
          frame "DATALOG5" {
            w765 = T14 2 items=["no dialog", "OK message", "continue or stop message", "OK message + warnings", "continue/stop + warnings"] ("type of dialog (OK msg:1)")
            # "datalog of OP 50"
            n301 = call "PADMINI_AUTO_BARCODE_STRING 50.vi"("Enum"=enum16{"Read", "Write"}."Read", "error in (no error)"=w758) -> ("error out"=w760:errorcluster, "Input 2"=w754:string[])  [unwired: 8 in]
            n302 = call "PADMINI_AUTO_CYCLE VALUE 50.vi"("Enum"=enum16{"Read", "Write"}."Read", "error in (no error)"=w758) -> ("Input 2"=w756:sgl[])  [unwired: 8 in, 1 out]
            n303 = Number To Fractional String(number=w756, precision (6)=i16 2) -> (F-format string=w755:string[])  [unwired: 2 in]
            n304 = case shown="False" w770 {
              tunnel: w771 -> [w792 w814]
              tunnel: w760 -> [w793 w813]
              tunnel: [w796 w812] -> w768
              tunnel: [w795 w811] -> w766
              tunnel: w769 -> [w791 _]
              tunnel: w755 -> [w787 w798]
              tunnel: w754 -> [w782 w797]
              frame False {
                # "DO TRACEBILITY"
                n305 = Index Array(array=w782) -> (element #1=w783:string, element #2=w779:string, element #3=w778:string, element #4=w777:string, element #5=w775:string)  [unwired: 5 in]
                n306 = local read "SHIFT"() -> (w794:string)
                n307 = Index Array(array=w787) -> (element #1=w786:string, element #2=w781:string, element #3=w780:string)  [unwired: 3 in]
                n308 = call <vilib>:"Trim Whitespace.vi"("string"=w783) -> ("trimmed string"=w784:string)  [unwired: 1 in]
                n309 = call "PADMINI_SHIFT_DATE.vi"("SHIFT"=w794) -> ("date/time string"=w776:string)  [unwired: 10 in]
                n310 = Format Into String(format string="Where BARCODE='%s' ", w784) -> (resulting string=w789:string)  [unwired: 2 in, 1 out]
                n311 = Bundle("date/time string"=w776, "Input 2"=w786, "Input 2"=w779, "Input 2"=w781, "Input 2"=w778, "Input 2"=w780, "Input 2"=w777, "Input 2"=w775) -> (w785:T23)  [unwired: 1 in]
                n312 = call <vilib>:"DB Tools Update Data.vi"("condition"=w789, "data"=w785, "error in (no error)"=w793, "columns"=string[] ["OP50_DATE", "OP50_NUT_TORQUE", "OP50_NUT_STATUS", "OP50_RH_STATUS", "OP50_RH_MOTOR_SCREW", "OP50_LH_STATUS", "OP50_LH_MOTOR_SCREW", "OP50_FINAL_RST"], "table"=w791, "connection reference"=w792) -> ("error out"=w795:errorcluster, "connection reference out"=w796:T13)  [unwired: 4 in]
              }
              frame True {
                # "TRAC BYPASS"
                n313 = local read "SHIFT"() -> (w799:string)
                n314 = Index Array(array=w797) -> (element #2=w803:string, element #3=w802:string, element #4=w807:string)  [unwired: 4 in, 1 out]
                n315 = Index Array(array=w798) -> (element #1=w806:string, element #2=w805:string, element #3=w804:string)  [unwired: 3 in]
                n316 = call "PADMINI_SHIFT_DATE.vi"("SHIFT"=w799) -> ("date/time string"=w800:string)  [unwired: 10 in]
                n317 = Bundle("date/time string"=w800, "SHIFT"=w799, "Input 2"=w806, "Input 2"=w803, "Input 2"=w805, "Input 2"=w802, "Input 2"=w804, "Input 2"=w807) -> (w801:T24)  [unwired: 1 in]
                n318 = To Variant(anything=w801) -> (Variant=w810:variant)
                n319 = call <vilib>:"DB Tools Insert Data.vi"("data"=w810, "error in (no error)"=w813, "columns"=string[] ["DATE", "SHIFT", "ST5_SCREW1_DATA", "ST5_SCREW1_STATUS", "ST5_SCREW2_DATA", "ST5_SCREW2_STATUS", "ST5_SCREW3_DATA", "ST5_FINAL_RST"], "table"="ST5_REPORT", "connection reference"=w814) -> ("error out"=w811:errorcluster, "connection reference out"=w812:T13)  [unwired: 5 in]
              }
            }
            n320 = call <vilib>:"Simple Error Handler.vi"("type of dialog (OK msg:1)"=w765, "error in (no error)"=w766) -> ("error out"=w764:errorcluster)  [unwired: 3 in, 4 out]
            n321 = call <vilib>:"Clear Errors.vi"("error in (no error)"=w764) -> ("error out"=w762:errorcluster)  [unwired: 5 in, 1 out]
            n322 = flat-sequence {
              tunnel: [w774] -> w753
              tunnel: w762 -> [w774]
              frame #0 {
                # "UPDATE op 20 save"
                n323 = global write "DATA LOG.vi" "OP 50 reset"(TRUE) -> ()
              }
            }
          }
          frame "SCAN6" {
            # "STATION OP 60"
            n324 = case shown="False" w821 {
              tunnel: w825 -> [w846 w852]
              tunnel: w824 -> [w839 w851]
              tunnel: w823 -> [_ _]
              tunnel: [w841 w850] -> w820
              tunnel: [w840 w852] -> w822
              tunnel: [w831 "" ("trimmed string")] -> _
              frame False {
                n325 = call "PADMINI_AUTO_BARCODE_STRING 60.vi"("Enum"=enum16{"Read", "Write"}."Read", "error in (no error)"=w839) -> ("error out"=w838:errorcluster, "Input 2"=w833:string[])  [unwired: 8 in]
                n326 = Index Array(array=w833) -> (element=w832:string)  [unwired: 1 in]
                n327 = call <vilib>:"Trim Whitespace.vi"("string"=w832) -> ("trimmed string"=w831:string)  [unwired: 1 in]
                n328 = Format Into String(format string="WHERE BARCODE  ='%s'", w831) -> (resulting string=w834:string)  [unwired: 2 in, 1 out]
                n329 = call <vilib>:"DB Tools Select Data.vi"("condition"=w834, "error in (no error)"=w838, "columns"=string[] ["BARCODE", "OP50_FINAL_RST", "OP60_FINAL_RST"], "table"="REPORT", "connection reference"=w846) -> ("error out"=w844:errorcluster, "data"=w843:variant[][], "connection reference out"=w840:T13)  [unwired: 1 in]
                n330 = call "PADMINI_varient_to_data.vi"("error in (no error)"=w844, "data"=w843) -> ("error out"=w842:errorcluster, "Array"=w828:string[][])  [unwired: 8 in]
                n331 = Index Array(array=w828, index (row)=0 ("disabled index (col)")) -> (element=→"SCAN OP60":string[])  [unwired: 1 in]
                n332 = call "RESPONSE_LOGIC.vi"("Array"=w828) -> ("Not Found"=w826:i32[])  [unwired: 10 in]
                "OP60 STATUS" <- w826
                n333 = call "PADMINI_AUTO_BARCODE_STATUS 60.vi"("Enum"=enum16{"Read", "Write"}."Write", "error in (no error)"=w842, "I/P"=w826) -> ("error out"=w841:errorcluster)  [unwired: 7 in, 1 out]
              }
              frame True {
                w847 = i32[] [0, 0, 0, 0, 0]  # I/P
                n334 = call "PADMINI_AUTO_BARCODE_STATUS 60.vi"("Enum"=enum16{"Read", "Write"}."Write", "error in (no error)"=w851, "I/P"=w847) -> ("error out"=w850:errorcluster)  [unwired: 7 in, 1 out]
              }
            }
            n335 = flat-sequence {
              tunnel: [w854] -> w819
              tunnel: w820 -> [w854]
              frame #0 {
                # "UPDATE op 60 SCAN sTATUS"
                n336 = global write "DATA LOG.vi" "OP 60 Outputs"(TRUE) -> ()
              }
            }
          }
          frame "DATALOG6" {
            w868 = T14 2 items=["no dialog", "OK message", "continue or stop message", "OK message + warnings", "continue/stop + warnings"] ("type of dialog (OK msg:1)")
            # "datalog of OP 60"
            n337 = call "PADMINI_AUTO_BARCODE_STRING 60.vi"("Enum"=enum16{"Read", "Write"}."Read", "error in (no error)"=w860) -> ("error out"=w862:errorcluster, "Input 2"=w856:string[])  [unwired: 8 in]
            n338 = call "PADMINI_AUTO_CYCLE VALUE 60.vi"("Enum"=enum16{"Read", "Write"}."Read", "error in (no error)"=w860) -> ("Input 2"=w858:sgl[])  [unwired: 8 in, 1 out]
            n339 = Number To Fractional String(number=w858, precision (6)=i16 2) -> (F-format string=w857:string[])  [unwired: 2 in]
            n340 = case shown="False" w873 {
              tunnel: w874 -> [w901 w929]
              tunnel: w862 -> [w902 w928]
              tunnel: [w905 w927] -> w871
              tunnel: [w904 w926] -> w869
              tunnel: w872 -> [w900 _]
              tunnel: w857 -> [w896 w909]
              tunnel: w856 -> [w892 w908]
              frame False {
                # "DO TRACEBILITY"
                n341 = Index Array(array=w892) -> (element #1=w893:string, element #2=w884:string, element #3=w883:string, element #4=w882:string, element #5=w881:string, element #6=w880:string, element #7=w879:string, element #8=w878:string)  [unwired: 8 in]
                n342 = local read "SHIFT"() -> (w903:string)
                n343 = Index Array(array=w896) -> (element #1=w890:string, element #2=w889:string, element #3=w888:string, element #4=w887:string, element #5=w886:string, element #6=w885:string)  [unwired: 6 in]
                n344 = call <vilib>:"Trim Whitespace.vi"("string"=w893) -> ("trimmed string"=w894:string)  [unwired: 1 in]
                n345 = call "PADMINI_SHIFT_DATE.vi"("SHIFT"=w903) -> ("date/time string"=w891:string)  [unwired: 10 in]
                n346 = Format Into String(format string="Where BARCODE='%s' ", w894) -> (resulting string=w898:string)  [unwired: 2 in, 1 out]
                n347 = Bundle("date/time string"=w891, "Input 2"=w890, "Input 2"=w884, "Input 2"=w889, "Input 2"=w883, "Input 2"=w888, "Input 2"=w882, "Input 2"=w887, "Input 2"=w881, "Input 2"=w886, "Input 2"=w880, "Input 2"=w885, "Input 2"=w879, "Input 2"=w878) -> (w895:T25)  [unwired: 1 in]
                n348 = call <vilib>:"DB Tools Update Data.vi"("condition"=w898, "data"=w895, "error in (no error)"=w902, "columns"=string[] ["OP60_DATE", "OP60_SCREW1_DATA", "OP60_SCREW1_STATUS", "OP60_SCREW2_DATA", "OP60_SCREW2_STATUS", "OP60_SCREW3_DATA", "OP60_SCREW3_STATUS", "OP60_SCREW4_DATA", "OP60_SCREW4_STATUS", "OP60_SCREW5_DATA", "OP60_SCREW5_STATUS", "OP60_SCREW6_DATA", "OP60_SCREW6_STATUS", "OP60_FINAL_RST"], "table"=w900, "connection reference"=w901) -> ("error out"=w904:errorcluster, "connection reference out"=w905:T13)  [unwired: 4 in]
              }
              frame True {
                # "TRAC BYPASS"
                n349 = local read "SHIFT"() -> (w906:string)
                n350 = call "PADMINI_SHIFT_DATE.vi"("SHIFT"=w906) -> ("date/time string"=w907:string)  [unwired: 10 in]
                n351 = Index Array(array=w908) -> (element #2=w917:string, element #3=w916:string, element #4=w915:string, element #5=w913:string, element #6=w921:string, element #7=w922:string)  [unwired: 7 in, 1 out]
                n352 = Index Array(array=w909) -> (element #1=w920:string, element #2=w919:string, element #3=w918:string, element #4=w914:string, element #5=w912:string, element #6=w911:string)  [unwired: 6 in]
                n353 = Bundle("date/time string"=w907, "SHIFT"=w906, "Input 2"=w920, "Input 2"=w917, "Input 2"=w919, "Input 2"=w916, "Input 2"=w918, "Input 2"=w915, "Input 2"=w914, "Input 2"=w913, "Input 2"=w912, "Input 2"=w911, "Input 2"=w921, "Input 2"=w922) -> (w910:T26)  [unwired: 1 in]
                n354 = To Variant(anything=w910) -> (Variant=w925:variant)
                n355 = call <vilib>:"DB Tools Insert Data.vi"("data"=w925, "error in (no error)"=w928, "columns"=string[] ["DATE", "SHIFT", "ST6_SCREW1_DATA", "ST6_SCREW1_STATUS", "ST6_SCREW2_DATA", "ST6_SCREW2_STATUS", "ST6_SCREW3_DATA", "ST6_SCREW3_STATUS", "ST6_SCREW4_DATA", "ST6_SCREW4_STATUS", "ST6_SCREW5_DATA", "ST6_SCREW5_STATUS", "ST6_SCREW6_DATA", "ST6_SCREW6_STATUS", "ST6_FINAL_RST"], "table"="ST6_REPORT", "connection reference"=w929) -> ("error out"=w926:errorcluster, "connection reference out"=w927:T13)  [unwired: 5 in]
              }
            }
            n356 = call <vilib>:"Simple Error Handler.vi"("type of dialog (OK msg:1)"=w868, "error in (no error)"=w869) -> ("error out"=w867:errorcluster)  [unwired: 3 in, 4 out]
            n357 = call <vilib>:"Clear Errors.vi"("error in (no error)"=w867) -> ("error out"=w865:errorcluster)  [unwired: 5 in, 1 out]
            n358 = flat-sequence {
              tunnel: [w877] -> w855
              tunnel: w865 -> [w877]
              frame #0 {
                # "UPDATE op 20 save"
                n359 = global write "DATA LOG.vi" "OP 60 reset"(TRUE) -> ()
              }
            }
          }
          frame "SCAN7" {
            # "STATION OP 70"
            n360 = case shown="False" w936 {
              tunnel: w940 -> [w961 w967]
              tunnel: w939 -> [w954 w966]
              tunnel: w938 -> [w946 _]
              tunnel: [w956 w965] -> w935
              tunnel: [w955 w967] -> w937
              tunnel: [w947 "" ("trimmed string")] -> _
              frame False {
                n361 = call "PADMINI_AUTO_BARCODE_STRING 70.vi"("Enum"=enum16{"Read", "Write"}."Read", "error in (no error)"=w954) -> ("error out"=w953:errorcluster, "Input 2"=w949:string[])  [unwired: 8 in]
                n362 = Index Array(array=w949) -> (element=w948:string)  [unwired: 1 in]
                n363 = call <vilib>:"Trim Whitespace.vi"("string"=w948) -> ("trimmed string"=w947:string)  [unwired: 1 in]
                n364 = Format Into String(format string="WHERE BARCODE  ='%s'", w947) -> (resulting string=w950:string)  [unwired: 2 in, 1 out]
                n365 = call <vilib>:"DB Tools Select Data.vi"("condition"=w950, "error in (no error)"=w953, "columns"=string[] ["BARCODE", "OP60_FINAL_RST", "OP70_FINAL_RST"], "table"=w946, "connection reference"=w961) -> ("error out"=w959:errorcluster, "data"=w958:variant[][], "connection reference out"=w955:T13)  [unwired: 1 in]
                n366 = call "PADMINI_varient_to_data.vi"("error in (no error)"=w959, "data"=w958) -> ("error out"=w957:errorcluster, "Array"=w943:string[][])  [unwired: 8 in]
                n367 = Index Array(array=w943, index (row)=0 ("disabled index (col)")) -> (element=→"SCAN OP70":string[])  [unwired: 1 in]
                n368 = call "RESPONSE_LOGIC.vi"("Array"=w943) -> ("Not Found"=w941:i32[])  [unwired: 10 in]
                "OP70 STATUS" <- w941
                n369 = call "PADMINI_AUTO_BARCODE_STATUS 70.vi"("Enum"=enum16{"Read", "Write"}."Write", "error in (no error)"=w957, "I/P"=w941) -> ("error out"=w956:errorcluster)  [unwired: 7 in, 1 out]
              }
              frame True {
                w962 = i32[] [0, 0, 0, 0, 0]  # I/P
                n370 = call "PADMINI_AUTO_BARCODE_STATUS 70.vi"("Enum"=enum16{"Read", "Write"}."Write", "error in (no error)"=w966, "I/P"=w962) -> ("error out"=w965:errorcluster)  [unwired: 7 in, 1 out]
              }
            }
            n371 = flat-sequence {
              tunnel: [w969] -> w934
              tunnel: w935 -> [w969]
              frame #0 {
                # "UPDATE op 70 SCAN sTATUS"
                n372 = global write "DATA LOG.vi" "OP 70 Outputs"(TRUE) -> ()
              }
            }
          }
          frame "DATALOG7" {
            w983 = T14 2 items=["no dialog", "OK message", "continue or stop message", "OK message + warnings", "continue/stop + warnings"] ("type of dialog (OK msg:1)")
            # "datalog of OP 70"
            n373 = call "PADMINI_AUTO_BARCODE_STRING 70.vi"("Enum"=enum16{"Read", "Write"}."Read", "error in (no error)"=w975) -> ("error out"=w977:errorcluster, "Input 2"=w971:string[])  [unwired: 8 in]
            n374 = call "PADMINI_AUTO_CYCLE VALUE 70.vi"("Enum"=enum16{"Read", "Write"}."Read", "error in (no error)"=w975) -> ("Input 2"=w973:sgl[])  [unwired: 8 in, 1 out]
            n375 = Number To Fractional String(number=w973, precision (6)=i16 4) -> (F-format string=w972:string[])  [unwired: 2 in]
            n376 = case shown="False" w988 {
              tunnel: w989 -> [w1007 w1025]
              tunnel: w977 -> [w1008 w1024]
              tunnel: [w1010 w1023] -> w986
              tunnel: [w1009 w1022] -> w984
              tunnel: w987 -> [w1006 _]
              tunnel: w972 -> [w1002 w1012]
              tunnel: w971 -> [w997 w1011]
              frame False {
                # "DO TRACEBILITY"
                n377 = Index Array(array=w997) -> (element #1=w998:string, element #2=w996:string)  [unwired: 2 in]
                n378 = call <vilib>:"Trim Whitespace.vi"("string"=w998) -> ("trimmed string"=w999:string)  [unwired: 1 in]
                n379 = local read "SHIFT"() -> (w994:string)
                n380 = Index Array(array=w1002) -> (element #1=w1001:string, element #2=w995:string)  [unwired: 2 in]
                n381 = call "PADMINI_SHIFT_DATE.vi"("SHIFT"=w994) -> ("date/time string"=w993:string)  [unwired: 10 in]
                n382 = Bundle("date/time string"=w993, "Input 2"=w1001, "Input 2"=w995, "Input 2"=w996) -> (w1000:T27)  [unwired: 1 in]
                n383 = Format Into String(format string="Where BARCODE='%s' ", w999) -> (resulting string=w1004:string)  [unwired: 2 in, 1 out]
                n384 = call <vilib>:"DB Tools Update Data.vi"("condition"=w1004, "data"=w1000, "error in (no error)"=w1008, "columns"=string[] ["OP70_DATE", "OP70_FULL_OPEN", "OP70_FULL_CLOSE", "OP70_FINAL_RST"], "table"=w1006, "connection reference"=w1007) -> ("error out"=w1009:errorcluster, "connection reference out"=w1010:T13)  [unwired: 4 in]
              }
              frame True {
                # "TRAC BYPASS"
                n385 = local read "SHIFT"() -> (w1013:string)
                n386 = call "PADMINI_SHIFT_DATE.vi"("SHIFT"=w1013) -> ("date/time string"=w1014:string)  [unwired: 10 in]
                n387 = Index Array(array=w1011) -> (element #2=w1017:string)  [unwired: 2 in, 1 out]
                n388 = Index Array(array=w1012) -> (element #1=w1018:string, element #2=w1016:string)  [unwired: 2 in]
                n389 = Bundle("date/time string"=w1014, "SHIFT"=w1013, "Input 2"=w1018, "Input 2"=w1016, "Input 2"=w1017) -> (w1015:T28)  [unwired: 1 in]
                n390 = To Variant(anything=w1015) -> (Variant=w1021:variant)
                n391 = call <vilib>:"DB Tools Insert Data.vi"("data"=w1021, "error in (no error)"=w1024, "columns"=string[] ["DATE_OP70", "SHIFT", "OP70_FULL_OPEN", "OP70_FULL_CLOSE", "OP70_FINAL_RST"], "table"="ST7_REPORT", "connection reference"=w1025) -> ("error out"=w1022:errorcluster, "connection reference out"=w1023:T13)  [unwired: 5 in]
              }
            }
            n392 = call <vilib>:"Simple Error Handler.vi"("type of dialog (OK msg:1)"=w983, "error in (no error)"=w984) -> ("error out"=w982:errorcluster)  [unwired: 3 in, 4 out]
            n393 = call <vilib>:"Clear Errors.vi"("error in (no error)"=w982) -> ("error out"=w980:errorcluster)  [unwired: 5 in, 1 out]
            n394 = flat-sequence {
              tunnel: [w992] -> w970
              tunnel: w980 -> [w992]
              frame #0 {
                # "UPDATE op 20 save"
                n395 = global write "DATA LOG.vi" "OP 70 reset"(TRUE) -> ()
              }
            }
          }
          frame "SCAN8" {
            # "STATION OP 80"
            n396 = case shown="False" w1032 {
              tunnel: w1036 -> [w1057 w1063]
              tunnel: w1035 -> [w1050 w1062]
              tunnel: w1034 -> [w1042 _]
              tunnel: [w1052 w1061] -> w1031
              tunnel: [w1051 w1063] -> w1033
              tunnel: [w1043 "" ("trimmed string")] -> _
              frame False {
                (unwired) "REPORT"
                n397 = call "PADMINI_AUTO_BARCODE_STRING 80.vi"("Enum"=enum16{"Read", "Write"}."Read", "error in (no error)"=w1050) -> ("error out"=w1049:errorcluster, "Input 2"=w1045:string[])  [unwired: 8 in]
                n398 = Index Array(array=w1045) -> (element=w1044:string)  [unwired: 1 in]
                n399 = call <vilib>:"Trim Whitespace.vi"("string"=w1044) -> ("trimmed string"=w1043:string)  [unwired: 1 in]
                n400 = Format Into String(format string="WHERE BARCODE  ='%s'", w1043) -> (resulting string=w1046:string)  [unwired: 2 in, 1 out]
                n401 = call <vilib>:"DB Tools Select Data.vi"("condition"=w1046, "error in (no error)"=w1049, "columns"=string[] ["BARCODE", "OP70_FINAL_RST", "OP80_FINAL_RST"], "table"=w1042, "connection reference"=w1057) -> ("error out"=w1055:errorcluster, "data"=w1054:variant[][], "connection reference out"=w1051:T13)  [unwired: 1 in]
                n402 = call "PADMINI_varient_to_data.vi"("error in (no error)"=w1055, "data"=w1054) -> ("error out"=w1053:errorcluster, "Array"=w1039:string[][])  [unwired: 8 in]
                n403 = Index Array(array=w1039, index (row)=0 ("disabled index (col)")) -> (element=→"SCAN OP80":string[])  [unwired: 1 in]
                n404 = call "RESPONSE_LOGIC.vi"("Array"=w1039) -> ("Not Found"=w1038:i32[])  [unwired: 10 in]
                "OP80 STATUS" <- w1038
                n405 = call "PADMINI_AUTO_BARCODE_STATUS 80.vi"("Enum"=enum16{"Read", "Write"}."Write", "error in (no error)"=w1053, "I/P"=w1038) -> ("error out"=w1052:errorcluster)  [unwired: 7 in, 1 out]
              }
              frame True {
                w1058 = i32[] [0, 0, 0, 0, 0]  # I/P
                n406 = call "PADMINI_AUTO_BARCODE_STATUS 80.vi"("Enum"=enum16{"Read", "Write"}."Write", "error in (no error)"=w1062, "I/P"=w1058) -> ("error out"=w1061:errorcluster)  [unwired: 7 in, 1 out]
              }
            }
            n407 = flat-sequence {
              tunnel: [w1065] -> w1030
              tunnel: w1031 -> [w1065]
              frame #0 {
                # "UPDATE op 80 SCAN sTATUS"
                n408 = global write "DATA LOG.vi" "OP 80 Outputs"(TRUE) -> ()
              }
            }
          }
          frame "DATALOG8" {
            w1079 = T14 2 items=["no dialog", "OK message", "continue or stop message", "OK message + warnings", "continue/stop + warnings"] ("type of dialog (OK msg:1)")
            # "datalog of OP 80"
            n409 = call "PADMINI_AUTO_BARCODE_STRING 80.vi"("Enum"=enum16{"Read", "Write"}."Read", "error in (no error)"=w1071) -> ("error out"=w1073:errorcluster, "Input 2"=w1067:string[])  [unwired: 8 in]
            n410 = call "PADMINI_AUTO_CYCLE VALUE 80.vi"("Enum"=enum16{"Read", "Write"}."Read", "error in (no error)"=w1071) -> ("Input 2"=w1069:sgl[])  [unwired: 8 in, 1 out]
            n411 = Number To Fractional String(number=w1069, precision (6)=i16 2) -> (F-format string=w1068:string[])  [unwired: 2 in]
            n412 = case shown="False" w1084 {
              tunnel: w1085 -> [w1103 w1121]
              tunnel: w1073 -> [w1104 w1120]
              tunnel: [w1106 w1119] -> w1082
              tunnel: [w1105 w1118] -> w1080
              tunnel: w1083 -> [w1102 _]
              tunnel: w1068 -> [w1098 w1109]
              tunnel: w1067 -> [w1094 w1110]
              frame False {
                # "DO TRACEBILITY"
                n413 = Index Array(array=w1094) -> (element #1=w1095:string, element #2=w1090:string, element #3=w1089:string)  [unwired: 3 in]
                n414 = call <vilib>:"Trim Whitespace.vi"("string"=w1095) -> ("trimmed string"=w1096:string)  [unwired: 1 in]
                n415 = local read "SHIFT"() -> (w1093:string)
                n416 = Index Array(array=w1098) -> (element=w1091:string)  [unwired: 1 in]
                n417 = call "PADMINI_SHIFT_DATE.vi"("SHIFT"=w1093) -> ("date/time string"=w1092:string)  [unwired: 10 in]
                n418 = Bundle("date/time string"=w1092, "Input 2"=w1090, "Input 2"=w1091, "Input 2"=w1089) -> (w1097:T27)  [unwired: 1 in]
                n419 = Format Into String(format string="Where BARCODE='%s' ", w1096) -> (resulting string=w1100:string)  [unwired: 2 in, 1 out]
                n420 = call <vilib>:"DB Tools Update Data.vi"("condition"=w1100, "data"=w1097, "error in (no error)"=w1104, "columns"=string[] ["OP80_DATE", "OP80_LOCTITE_STATUS", "OP80_PLUG_PRESS_LOA", "OP80_FINAL_RST"], "table"=w1102, "connection reference"=w1103) -> ("error out"=w1105:errorcluster, "connection reference out"=w1106:T13)  [unwired: 4 in]
              }
              frame True {
                # "TRAC BYPASS"
                n421 = local read "SHIFT"() -> (w1107:string)
                n422 = call "PADMINI_SHIFT_DATE.vi"("SHIFT"=w1107) -> ("date/time string"=w1108:string)  [unwired: 10 in]
                n423 = Index Array(array=w1110) -> (element #2=w1114:string, element #3=w1113:string)  [unwired: 3 in, 1 out]
                n424 = Index Array(array=w1109) -> (element=w1112:string)  [unwired: 1 in]
                n425 = Bundle("date/time string"=w1108, "SHIFT"=w1107, "Input 2"=w1112, "Input 2"=w1114, "Input 2"=w1113) -> (w1111:T28)  [unwired: 1 in]
                n426 = To Variant(anything=w1111) -> (Variant=w1117:variant)
                n427 = call <vilib>:"DB Tools Insert Data.vi"("data"=w1117, "error in (no error)"=w1120, "columns"=string[] ["DATE", "SHIFT", "ST8_DISPENSING", "ST8_LOAD", "ST8_FINAL_RST"], "table"="ST8_REPORT", "connection reference"=w1121) -> ("error out"=w1118:errorcluster, "connection reference out"=w1119:T13)  [unwired: 5 in]
              }
            }
            n428 = call <vilib>:"Simple Error Handler.vi"("type of dialog (OK msg:1)"=w1079, "error in (no error)"=w1080) -> ("error out"=w1078:errorcluster)  [unwired: 3 in, 4 out]
            n429 = call <vilib>:"Clear Errors.vi"("error in (no error)"=w1078) -> ("error out"=w1076:errorcluster)  [unwired: 5 in, 1 out]
            n430 = flat-sequence {
              tunnel: [w1088] -> w1066
              tunnel: w1076 -> [w1088]
              frame #0 {
                # "UPDATE op 20 save"
                n431 = global write "DATA LOG.vi" "OP 80 reset"(TRUE) -> ()
              }
            }
          }
          frame "SCAN9" {
            # "STATION OP 90"
            n432 = case shown="False" w1128 {
              tunnel: w1132 -> [w1153 w1159]
              tunnel: w1131 -> [w1146 w1158]
              tunnel: w1130 -> [w1138 _]
              tunnel: [w1148 w1157] -> w1127
              tunnel: [w1147 w1159] -> w1129
              tunnel: [w1139 "" ("trimmed string")] -> _
              frame False {
                (unwired) "REPORT"
                n433 = call "PADMINI_AUTO_BARCODE_STRING 90.vi"("Enum"=enum16{"Read", "Write"}."Read", "error in (no error)"=w1146) -> ("error out"=w1145:errorcluster, "Input 2"=w1141:string[])  [unwired: 8 in]
                n434 = Index Array(array=w1141) -> (element=w1140:string)  [unwired: 1 in]
                n435 = call <vilib>:"Trim Whitespace.vi"("string"=w1140) -> ("trimmed string"=w1139:string)  [unwired: 1 in]
                n436 = Format Into String(format string="WHERE BARCODE  ='%s'", w1139) -> (resulting string=w1142:string)  [unwired: 2 in, 1 out]
                n437 = call <vilib>:"DB Tools Select Data.vi"("condition"=w1142, "error in (no error)"=w1145, "columns"=string[] ["BARCODE", "OP80_FINAL_RST", "OP90_FINAL_RST"], "table"=w1138, "connection reference"=w1153) -> ("error out"=w1151:errorcluster, "data"=w1150:variant[][], "connection reference out"=w1147:T13)  [unwired: 1 in]
                n438 = call "PADMINI_varient_to_data.vi"("error in (no error)"=w1151, "data"=w1150) -> ("error out"=w1149:errorcluster, "Array"=w1135:string[][])  [unwired: 8 in]
                n439 = Index Array(array=w1135, index (row)=0 ("disabled index (col)")) -> (element=→"SCAN OP90":string[])  [unwired: 1 in]
                n440 = call "RESPONSE_LOGIC.vi"("Array"=w1135) -> ("Not Found"=w1133:i32[])  [unwired: 10 in]
                "OP90 STATUS" <- w1133
                n441 = call "PADMINI_AUTO_BARCODE_STATUS 90.vi"("Enum"=enum16{"Read", "Write"}."Write", "error in (no error)"=w1149, "I/P"=w1133) -> ("error out"=w1148:errorcluster)  [unwired: 7 in, 1 out]
              }
              frame True {
                w1154 = i32[] [0, 0, 0, 0, 0]  # I/P
                n442 = call "PADMINI_AUTO_BARCODE_STATUS 90.vi"("Enum"=enum16{"Read", "Write"}."Write", "error in (no error)"=w1158, "I/P"=w1154) -> ("error out"=w1157:errorcluster)  [unwired: 7 in, 1 out]
              }
            }
            n443 = flat-sequence {
              tunnel: [w1161] -> w1126
              tunnel: w1127 -> [w1161]
              frame #0 {
                # "UPDATE op 90 SCAN sTATUS"
                n444 = global write "DATA LOG.vi" "OP 90 Outputs"(TRUE) -> ()
              }
            }
          }
          frame "DATALOG9" {
            w1175 = T14 2 items=["no dialog", "OK message", "continue or stop message", "OK message + warnings", "continue/stop + warnings"] ("type of dialog (OK msg:1)")
            # "datalog of OP 90"
            n445 = call "PADMINI_AUTO_BARCODE_STRING 90.vi"("Enum"=enum16{"Read", "Write"}."Read", "error in (no error)"=w1167) -> ("error out"=w1169:errorcluster, "Input 2"=w1164:string[])  [unwired: 8 in]
            n446 = call "PADMINI_AUTO_CYCLE VALUE 90.vi"("Enum"=enum16{"Read", "Write"}."Read", "error in (no error)"=w1167) -> ("Input 2"=w1163:sgl[])  [unwired: 8 in, 1 out]
            n447 = Number To Fractional String(number=w1163, precision (6)=i16 2) -> (F-format string=w1165:string[])  [unwired: 2 in]
            n448 = case shown="False" w1180 {
              tunnel: w1181 -> [w1200 w1219]
              tunnel: w1169 -> [w1201 w1218]
              tunnel: [w1203 w1217] -> w1178
              tunnel: [w1202 w1216] -> w1176
              tunnel: w1179 -> [w1199 _]
              tunnel: w1165 -> [w1195 w1208]
              tunnel: w1164 -> [w1191 w1207]
              frame False {
                # "DO TRACEBILITY"
                n449 = Index Array(array=w1191) -> (element #1=w1192:string, element #2=w1189:string, element #3=w1187:string)  [unwired: 3 in]
                n450 = call <vilib>:"Trim Whitespace.vi"("string"=w1192) -> ("trimmed string"=w1193:string)  [unwired: 1 in]
                n451 = local read "SHIFT"() -> (w1186:string)
                n452 = Index Array(array=w1195) -> (element #1=w1190:string, element #2=w1188:string)  [unwired: 2 in]
                n453 = call "PADMINI_SHIFT_DATE.vi"("SHIFT"=w1186) -> ("date/time string"=w1185:string)  [unwired: 10 in]
                n454 = Bundle("date/time string"=w1185, "Input 2"=w1190, "Input 2"=w1189, "Input 2"=w1188, "Input 2"=w1187) -> (w1194:T19)  [unwired: 1 in]
                n455 = Format Into String(format string="Where BARCODE='%s' ", w1193) -> (resulting string=w1197:string)  [unwired: 2 in, 1 out]
                n456 = call <vilib>:"DB Tools Update Data.vi"("condition"=w1197, "data"=w1194, "error in (no error)"=w1201, "columns"=string[] ["OP90_DATE", "OP90_SEAT_LEAK", "OP90_SEAT_STATUS", "OP90_STEAM_LEAK", "OP90_FINAL_RST"], "table"=w1199, "connection reference"=w1200) -> ("error out"=w1202:errorcluster, "connection reference out"=w1203:T13)  [unwired: 4 in]
              }
              frame True {
                # "TRAC BYPASS"
                n457 = local read "SHIFT"() -> (w1204:string)
                n458 = call "PADMINI_SHIFT_DATE.vi"("SHIFT"=w1204) -> ("date/time string"=w1205:string)  [unwired: 10 in]
                n459 = Index Array(array=w1207) -> (element #2=w1212:string, element #3=w1210:string)  [unwired: 3 in, 1 out]
                n460 = Index Array(array=w1208) -> (element #1=w1213:string, element #2=w1211:string)  [unwired: 2 in]
                n461 = Bundle("date/time string"=w1205, "SHIFT"=w1204, "Input 2"=w1213, "Input 2"=w1212, "Input 2"=w1211, "Input 2"=w1210) -> (w1209:T20)  [unwired: 1 in]
                n462 = To Variant(anything=w1209) -> (Variant=w1215:variant)
                n463 = call <vilib>:"DB Tools Insert Data.vi"("data"=w1215, "error in (no error)"=w1218, "columns"=string[] ["DATE", "SHIFT", "ST9_SEAT_LT_DATA", "ST9_SEAT_STATUS", "ST9_STEAM_LT_DATA", "ST9_FINAL_RST"], "table"="ST9_REPORT", "connection reference"=w1219) -> ("error out"=w1216:errorcluster, "connection reference out"=w1217:T13)  [unwired: 5 in]
              }
            }
            n464 = call <vilib>:"Simple Error Handler.vi"("type of dialog (OK msg:1)"=w1175, "error in (no error)"=w1176) -> ("error out"=w1174:errorcluster)  [unwired: 3 in, 4 out]
            n465 = call <vilib>:"Clear Errors.vi"("error in (no error)"=w1174) -> ("error out"=w1172:errorcluster)  [unwired: 5 in, 1 out]
            n466 = flat-sequence {
              tunnel: [w1184] -> w1162
              tunnel: w1172 -> [w1184]
              frame #0 {
                # "UPDATE op 20 save"
                n467 = global write "DATA LOG.vi" "OP 90 reset"(TRUE) -> ()
              }
            }
          }
          frame "SCAN10" {
            # "STATION OP 10"
            n468 = case shown="False" w1226 {
              tunnel: w1230 -> [w1251 w1257]
              tunnel: w1229 -> [w1245 w1256]
              tunnel: w1228 -> [w1237 _]
              tunnel: [w1235 w1255] -> w1225
              tunnel: [w1246 w1257] -> w1227
              tunnel: [w1238 "" ("trimmed string")] -> _
              frame False {
                (unwired) "REPORT"
                n469 = call "PADMINI_AUTO_BARCODE_STRING 100.vi"("Enum"=enum16{"Read", "Write"}."Read", "error in (no error)"=w1245) -> ("error out"=w1244:errorcluster, "Input 2"=w1240:string[])  [unwired: 8 in]
                n470 = Index Array(array=w1240) -> (element=w1239:string)  [unwired: 1 in]
                n471 = call <vilib>:"Trim Whitespace.vi"("string"=w1239) -> ("trimmed string"=w1238:string)  [unwired: 1 in]
                n472 = Format Into String(format string="WHERE BARCODE  ='%s'", w1238) -> (resulting string=w1241:string)  [unwired: 2 in, 1 out]
                n473 = call <vilib>:"DB Tools Select Data.vi"("condition"=w1241, "error in (no error)"=w1244, "columns"=string[] ["BARCODE", "OP90_FINAL_RST", "OP100_FINAL_RST"], "table"=w1237, "connection reference"=w1251) -> ("error out"=w1249:errorcluster, "data"=w1248:variant[][], "connection reference out"=w1246:T13)  [unwired: 1 in]
                n474 = call "PADMINI_varient_to_data.vi"("error in (no error)"=w1249, "data"=w1248) -> ("error out"=w1247:errorcluster, "Array"=w1233:string[][])  [unwired: 8 in]
                n475 = Index Array(array=w1233, index (row)=0 ("disabled index (col)")) -> (element=→"SCAN OP100":string[])  [unwired: 1 in]
                n476 = call "RESPONSE_LOGIC.vi"("Array"=w1233) -> ("Not Found"=w1231:i32[])  [unwired: 10 in]
                "OP100 STATUS" <- w1231
                n477 = call "PADMINI_AUTO_BARCODE_STATUS 100.vi"("Enum"=enum16{"Read", "Write"}."Write", "error in (no error)"=w1247, "I/P"=w1231) -> ("error out"=w1235:errorcluster)  [unwired: 7 in, 1 out]
              }
              frame True {
                w1252 = i32[] [0, 0, 0, 0, 0]  # I/P
                n478 = call "PADMINI_AUTO_BARCODE_STATUS 100.vi"("Enum"=enum16{"Read", "Write"}."Write", "error in (no error)"=w1256, "I/P"=w1252) -> ("error out"=w1255:errorcluster)  [unwired: 7 in, 1 out]
              }
            }
            n479 = flat-sequence {
              tunnel: [w1259] -> w1224
              tunnel: w1225 -> [w1259]
              frame #0 {
                # "UPDATE op 100 SCAN sTATUS"
                n480 = global write "DATA LOG.vi" "OP 100 Outputs"(TRUE) -> ()
              }
            }
          }
          frame "SCAN11" {
            # "STATION OP 110"
            n481 = case shown="False" w1266 {
              tunnel: w1270 -> [w1297 w1307]
              tunnel: w1269 -> [w1290 w1306]
              tunnel: w1268 -> [w1282 _]
              tunnel: [w1292 w1305] -> w1265
              tunnel: [w1291 w1307] -> w1267
              frame False {
                (unwired) "REPORT"
                # "OP100 OK\nOP 100 NG"
                n482 = call "PADMINI_AUTO_BARCODE_STRING 100.vi"("Enum"=enum16{"Read", "Write"}."Read", "error in (no error)"=w1290) -> ("error out"=w1289:errorcluster, "Input 2"=w1284:string[])  [unwired: 8 in]
                n483 = Index Array(array=w1284) -> (element=w1283:string)  [unwired: 1 in]
                n484 = call <vilib>:"Trim Whitespace.vi"("string"=w1283) -> ("trimmed string"=w1285:string)  [unwired: 1 in]
                n485 = Format Into String(format string="WHERE BARCODE  ='%s'", w1285) -> (resulting string=w1286:string)  [unwired: 2 in, 1 out]
                n486 = call <vilib>:"DB Tools Select Data.vi"("condition"=w1286, "error in (no error)"=w1289, "columns"=string[] ["BARCODE", "OP100_FINAL_RST"], "table"=w1282, "connection reference"=w1297) -> ("error out"=w1295:errorcluster, "data"=w1294:variant[][], "connection reference out"=w1291:T13)  [unwired: 1 in]
                n487 = call "PADMINI_varient_to_data.vi"("error in (no error)"=w1295, "data"=w1294) -> ("error out"=w1293:errorcluster, "Array"=w1273:string[][])  [unwired: 8 in]
                n488 = Index Array(array=w1273, index (row)=0 ("disabled index (col)")) -> (element=w1272:string[])  [unwired: 1 in]
                "SCAN OP110" <- w1272
                n489 = Index Array(array=w1272) -> (element #1=w1280:string, element #2=w1277:string)  [unwired: 2 in]
                n490 = Equal?(x="", y=w1280) -> (x = y?=w1279:bool)
                n491 = Equal?(x=w1277, y="OK") -> (x = y?=w1278:bool)
                n492 = case shown="True" w1279 {
                  tunnel: w1278 -> [w1298 _]
                  tunnel: [w1299 w1302] -> w1271
                  frame False {
                    # "BARCODE FOUND"
                    n493 = case shown="False" w1298 {
                      tunnel: [w1300 w1301] -> w1299
                      frame False {
                        w1300 = i32[] [0, 1]  # OK
                        # "CT ST REPEAT NG & EMPTY"
                      }
                      frame True {
                        w1301 = i32[] [1, 0]  # NG
                        # "CT ST REPEAT EMPTY"
                      }
                    }
                  }
                  frame True {
                    w1302 = i32[] [0, 1]  # Not Found
                    # "nO BARCODE FOUND"
                  }
                }
                "OP110 STATUS" <- w1271
                n494 = call "PADMINI_AUTO_BARCODE_STATUS 110.vi"("Enum"=enum16{"Read", "Write"}."Write", "error in (no error)"=w1293, "I/P"=w1271) -> ("error out"=w1292:errorcluster)  [unwired: 7 in, 1 out]
              }
              frame True {
                w1303 = i32[] [0, 0, 0, 0, 0]  # I/P
                n495 = call "PADMINI_AUTO_BARCODE_STATUS 100.vi"("Enum"=enum16{"Read", "Write"}."Write", "error in (no error)"=w1306, "I/P"=w1303) -> ("error out"=w1305:errorcluster)  [unwired: 7 in, 1 out]
              }
            }
            n496 = flat-sequence {
              tunnel: [w1309] -> w1264
              tunnel: w1265 -> [w1309]
              frame #0 {
                # "UPDATE op 100 SCAN sTATUS"
                n497 = global write "DATA LOG.vi" "OP 110 Outputs"(TRUE) -> ()
              }
            }
          }
          frame "DATALOG10" {
            w1323 = T14 2 items=["no dialog", "OK message", "continue or stop message", "OK message + warnings", "continue/stop + warnings"] ("type of dialog (OK msg:1)")
            # "datalog of OP 100"
            n498 = call "PADMINI_AUTO_BARCODE_STRING 100.vi"("Enum"=enum16{"Read", "Write"}."Read", "error in (no error)"=w1311) -> ("error out"=w1317:errorcluster, "Input 2"=w1313:string[])  [unwired: 8 in]
            n499 = call "PADMINI_AUTO_CYCLE VALUE 100.vi"("Enum"=enum16{"Read", "Write"}."Read", "error in (no error)"=w1311) -> ("Input 2"=w1312:sgl[])  [unwired: 8 in, 1 out]
            n500 = Number To Fractional String(number=w1312, precision (6)=i16 2) -> (F-format string=w1314:string[])  [unwired: 2 in]
            n501 = case shown="False" w1328 {
              tunnel: w1329 -> [w1356 w1381]
              tunnel: w1317 -> [w1357 w1380]
              tunnel: [w1359 w1379] -> w1326
              tunnel: [w1358 w1378] -> w1324
              tunnel: w1327 -> [w1355 _]
              tunnel: w1314 -> [w1351 w1363]
              tunnel: w1313 -> [w1348 w1364]
              frame False {
                # "DO TRACEBILITY"
                n502 = Index Array(array=w1348) -> (element #1=w1347:string, element #2=w1333:string)  [unwired: 2 in]
                n503 = call <vilib>:"Trim Whitespace.vi"("string"=w1347) -> ("trimmed string"=w1349:string)  [unwired: 1 in]
                n504 = Index Array(array=w1351) -> (element #1=w1344:string, element #2=w1343:string, element #3=w1342:string, element #4=w1341:string, element #5=w1340:string, element #6=w1339:string, element #7=w1338:string, element #8=w1337:string, element #9=w1336:string, element #10=w1335:string, element #11=w1334:string)  [unwired: 11 in]
                n505 = local read "SHIFT"() -> (w1346:string)
                n506 = call "PADMINI_SHIFT_DATE.vi"("SHIFT"=w1346) -> ("date/time string"=w1345:string)  [unwired: 10 in]
                n507 = Bundle("date/time string"=w1345, "Input 2"=w1344, "Input 2"=w1343, "Input 2"=w1342, "Input 2"=w1341, "Input 2"=w1340, "Input 2"=w1339, "Input 2"=w1338, "Input 2"=w1337, "Input 2"=w1336, "Input 2"=w1335, "Input 2"=w1334, "Input 2"=w1333) -> (w1350:T29)  [unwired: 1 in]
                n508 = Format Into String(format string="Where BARCODE='%s' ", w1349) -> (resulting string=w1353:string)  [unwired: 2 in, 1 out]
                n509 = call <vilib>:"DB Tools Update Data.vi"("condition"=w1353, "data"=w1350, "error in (no error)"=w1357, "columns"=string[] ["OP100_DATE", "OP100_SENSOR_OP_OPEN", "OP100_SENSOR_OP_CLOSE", "OP100_SENSOR_OP_FULL_CLOSE", "OP100_SENSOR_INITIAL", "OP100_MOTOR_START_OF_CLOSE", "OP100_MOTOR_FULL_CLOSE", "OP100_MOTOR_START_BACK", "OP100_MOTOR_FULL_OPEN", "OP100_RESPONSE_TIME_FWD", "OP100_RESPONSE_TIME_REV", "OP100_MOTOR_PEAK_CURRENT", "OP100_FINAL_RST"], "table"=w1355, "connection reference"=w1356) -> ("error out"=w1358:errorcluster, "connection reference out"=w1359:T13)  [unwired: 4 in]
              }
              frame True {
                # "TRAC BYPASS"
                n510 = local read "SHIFT"() -> (w1361:string)
                n511 = Index Array(array=w1364) -> (element=w1368:string)  [unwired: 1 in]
                n512 = call "PADMINI_SHIFT_DATE.vi"("SHIFT"=w1361) -> ("date/time string"=w1362:string)  [unwired: 10 in]
                n513 = Index Array(array=w1363) -> (element #1=w1374:string, element #2=w1373:string, element #3=w1360:string, element #4=w1366:string, element #5=w1372:string, element #6=w1367:string, element #7=w1371:string, element #8=w1370:string, element #9=w1369:string)  [unwired: 9 in]
                n514 = Bundle("date/time string"=w1362, "SHIFT"=w1361, "Input 2"=w1374, "Input 2"=w1373, "Input 2"=w1360, "Input 2"=w1360, "Input 2"=w1360, "Input 2"=w1366, "Input 2"=w1372, "Input 2"=w1367, "Input 2"=w1371, "Input 2"=w1370, "Input 2"=w1369, "Input 2"=w1368) -> (w1365:T26)  [unwired: 1 in]
                n515 = To Variant(anything=w1365) -> (Variant=w1377:variant)
                n516 = call <vilib>:"DB Tools Insert Data.vi"("data"=w1377, "error in (no error)"=w1380, "columns"=string[] ["DATE", "SHIFT", "ST10_SENSOR_OP_OPEN_V", "ST10_START_OF_CLOSE_SENSOR_V", "ST10_SENSOR_OP_FULL_CLOSE_V", "ST10_RESPONSE_TIME_FWD", "ST10_RESPONSE_TIME_REV", "ST10_MOTOR_V_START_OF_CLOSE_A", "ST10_MOTOR_V_FULL_CLOSE_B", "ST10_MOTOR_V_START_BACK_C", "ST10_MOTOR_V_FULL_OPEN_D", "ST10_MOTOR_RMS_CURRENT_A", "ST10_FINAL_RST"], "table"="ST10_REPORT", "connection reference"=w1381) -> ("error out"=w1378:errorcluster, "connection reference out"=w1379:T13)  [unwired: 5 in]
              }
            }
            n517 = call <vilib>:"Simple Error Handler.vi"("type of dialog (OK msg:1)"=w1323, "error in (no error)"=w1324) -> ("error out"=w1322:errorcluster)  [unwired: 3 in, 4 out]
            n518 = call <vilib>:"Clear Errors.vi"("error in (no error)"=w1322) -> ("error out"=w1320:errorcluster)  [unwired: 5 in, 1 out]
            n519 = flat-sequence {
              tunnel: [w1332] -> w1310
              tunnel: w1320 -> [w1332]
              frame #0 {
                # "UPDATE op 20 save"
                n520 = global write "DATA LOG.vi" "OP 100 reset"(TRUE) -> ()
              }
            }
          }
          frame "EMERGENCY STOP" {
          }
          frame "STOP" {
            n521 = global read "Global 1.vi" "BARCODE RECIPE"() -> (w1392:string)
            n522 = Bundle("BARCODE RECIPE"=w1392) -> (w1391:cluster{"BARCODE RECIPE":string})  [unwired: 1 in]
            n523 = call <vilib>:"DB Tools Update Data.vi"("data"=w1391, "error in (no error)"=w1397, "columns"=string[] ["PREVIOUS_LOADED_RECIPE"], "table"="BARCODE_RECIPE", "connection reference"=w1395) -> ("error out"=w1396:errorcluster, "connection reference out"=w1394:T13)  [unwired: 5 in]
          }
        }
      }
      frame Error {
        # "Return true in any case that should stop the loop."
      }
    }
    n524 = Unbundle By Name(w130) -> ("OP - 90"=→"OP - 90":T30, "OP - 100"=→"OP - 100":T10, "OP - 110"=→"OP - 110":cluster{"BARCODE":string})
    n525 = Unbundle By Name(w130) -> ("OP - 10"=→"OP - 10":T31, "OP - 20"=→"OP - 20":T5, "OP - 30"=→"OP - 30":T32, "OP - 40"=→"OP - 40":T2)
    n526 = Unbundle By Name(w130) -> ("OP - 50"=→"OP - 50":T1, "OP - 60"=→"OP - 60":T33, "OP - 70"=→"OP - 70":T34, "OP - 80"=→"OP - 80":T35)
    n527 = Wait (ms)(milliseconds to wait=u32 100) -> ()  [unwired: 1 out]
    n528 = call <vilib>:"Simple Error Handler.vi"("error in (no error)"=w124) -> ("error out"=w123:errorcluster)  [unwired: 4 in, 4 out]
  }
  n529 = while {
    shift-right: [w1421] -> w72
    shift-left: w22 -> [w1415]
    shift-right: [w1422] -> w66
    shift-left: w70 -> [w1430]
    stop <- w1420 stop-if-true
    n530 = local read "Shift_change"() -> (w1428:bool)
    n531 = call <vilib>:"Clear Errors.vi"("error in (no error)"=w1415) -> ("error out"=w1406:errorcluster)  [unwired: 5 in, 1 out]
    n532 = call "READ EMERGENCY BIT.vi"("Enum"=enum16{"Read", "Write"}."Read", "error in (no error)"=w1406) -> ("Array Out"=w1418:dbl[])  [unwired: 8 in, 1 out]
    n533 = case shown="True" w1428 {
      tunnel: w1406 -> [w1447 w1460]
      tunnel: [w1448 w1459] -> w1427
      frame False {
        n534 = local read "SHIFT_DATA 2"() -> (w1450:string[])
        n535 = Get Date/Time In Seconds() -> (seconds since 1Jan1904=w1449:timestamp)
        n536 = call "String To Time_4.vi"("error in (no error)"=w1447, "String Array In"=w1450) -> ("error out"=w1446:errorcluster, "Time Stamp Out"=w1445:timestamp[])  [unwired: 8 in]
        "Time Stamp Out 4" <- w1445
        n537 = call "Shift Calculation_4.vi"("error in (no error)"=w1446, "Current Time"=w1449, "Time Stamp Out"=w1445) -> ("error out"=w1444:errorcluster, "Shift"=w1443:i32)  [unwired: 7 in]
        n538 = call <vilib>:"Clear Errors.vi"("error in (no error)"=w1444) -> ()  [unwired: 5 in, 2 out]
        n539 = case shown="4" w1443 {
          tunnel: ["A" "B" "C" "D"] -> w1448
          frame 1, Default {
          }
          frame 2 {
          }
          frame 3 {
          }
          frame 4 {
          }
        }
      }
      frame True {
        n540 = local read "SHIFT_DATA"() -> (w1458:string[])
        n541 = Get Date/Time In Seconds() -> (seconds since 1Jan1904=w1461:timestamp)
        n542 = call "String To Time.vi"("error in (no error)"=w1460, "String Array In"=w1458) -> ("error out"=w1457:errorcluster, "Time Stamp Out"=w1462:timestamp[])  [unwired: 8 in]
        "Time Stamp Out" <- w1462
        n543 = call "Shift Calculation.vi"("error in (no error)"=w1457, "Current Time"=w1461, "Time Stamp Out"=w1462) -> ("error out"=w1456:errorcluster, "Shift"=w1455:i32)  [unwired: 7 in]
        "Shift 4" <- w1455
        n544 = call <vilib>:"Clear Errors.vi"("error in (no error)"=w1456) -> ()  [unwired: 5 in, 2 out]
        n545 = case shown="3" w1455 {
          tunnel: ["A" "B" "C"] -> w1459
          frame 1, Default {
          }
          frame 2 {
          }
          frame 3 {
          }
        }
      }
    }
    "SHIFT" <- w1427
    n546 = Index Array(array=w1418) -> (element=w1417:dbl)  [unwired: 1 in]
    n547 = call "VALUE_CHANGE - ST1_RESULT.vi"("Numeric"=w1417) -> ("Boolean"=w1416:bool)  [unwired: 9 in, 1 out]
    n548 = global write "Global 1.vi" "EMERGENCY STOP"(w1416) -> ()
    n549 = call "Trigger_Loggic.vi"("error in (no error)"=w1406) -> ("error out"=w1411:errorcluster, "Array"=w1431:i32[])  [unwired: 9 in]
    n550 = for {
      tunnel: w1431 -> [w1466] mode=indexing
      shift-right: [w1470] -> w1424
      shift-left: w1430 -> [w1469]
      shift-right: [w1468] -> w1423
      shift-left: w1411 -> [w1467]
      n551 = case shown="0" w1466 {
        tunnel: [w1473 w1478 w1482 w1488 w1493 w1498 w1503 w1508 w1513 w1518 w1523 w1528 w1533 w1538 w1543 w1548 w1553 w1558 w1563 w1568 w1573 w1578 w1583] -> w1470
        tunnel: w1469 -> [w1475 w1480 w1483 w1490 w1495 w1500 w1505 w1510 w1515 w1520 w1525 w1530 w1535 w1540 w1545 w1550 w1555 w1560 w1565 w1570 w1575 w1580 w1585]
        tunnel: [w1472 w1477 w1484 w1487 w1492 w1497 w1502 w1507 w1512 w1517 w1522 w1527 w1532 w1537 w1542 w1547 w1552 w1557 w1562 w1567 w1572 w1577 w1582] -> w1468
        tunnel: w1467 -> [w1474 w1479 w1485 w1489 w1494 w1499 w1504 w1509 w1514 w1519 w1524 w1529 w1534 w1539 w1544 w1549 w1554 w1559 w1564 w1569 w1574 w1579 w1584]
        frame -1, Default {
          # "DEFAULT"
          n552 = Enqueue Element(queue=w1475, element=cluster{"CASE 2":T12} {"CASE 2"=enum."-1"}, error in (no error)=w1474) -> (queue out=w1473:refnum<queue>, error out=w1472:errorcluster)  [unwired: 1 in, 1 out]
        }
        frame 0 {
          # "SCAN BARCODE OP 10"
          n553 = Enqueue Element(queue=w1480, element=cluster{"CASE 2":T12} {"CASE 2"=enum."-1"}, error in (no error)=w1479) -> (queue out=w1478:refnum<queue>, error out=w1477:errorcluster)  [unwired: 1 in, 1 out]
        }
        frame 1 {
          # "DATALOG OF OP 10"
          n554 = Enqueue Element(queue=w1483, element=cluster{"CASE 2":T12} {"CASE 2"=enum."SCAN1"}, error in (no error)=w1485) -> (queue out=w1482:refnum<queue>, error out=w1484:errorcluster)  [unwired: 1 in, 1 out]
        }
        frame 2 {
          # "SCAN BARCODE OP 20"
          n555 = Enqueue Element(queue=w1490, element=cluster{"CASE 2":T12} {"CASE 2"=enum."SCAN2"}, error in (no error)=w1489) -> (queue out=w1488:refnum<queue>, error out=w1487:errorcluster)  [unwired: 1 in, 1 out]
        }
        frame 3 {
          # "DATALOG OF OP 20"
          n556 = Enqueue Element(queue=w1495, element=cluster{"CASE 2":T12} {"CASE 2"=enum."DATALOG2"}, error in (no error)=w1494) -> (queue out=w1493:refnum<queue>, error out=w1492:errorcluster)  [unwired: 1 in, 1 out]
        }
        frame 4 {
          # "SCAN BARCODE OP 30"
          n557 = Enqueue Element(queue=w1500, element=cluster{"CASE 2":T12} {"CASE 2"=enum."SCAN3"}, error in (no error)=w1499) -> (queue out=w1498:refnum<queue>, error out=w1497:errorcluster)  [unwired: 1 in, 1 out]
        }
        frame 5 {
          # "DATALOG OF OP 30"
          n558 = Enqueue Element(queue=w1505, element=cluster{"CASE 2":T12} {"CASE 2"=enum."DATALOG3"}, error in (no error)=w1504) -> (queue out=w1503:refnum<queue>, error out=w1502:errorcluster)  [unwired: 1 in, 1 out]
        }
        frame 6 {
          # "SCAN BARCODE OP 40"
          n559 = Enqueue Element(queue=w1510, element=cluster{"CASE 2":T12} {"CASE 2"=enum."SCAN4"}, error in (no error)=w1509) -> (queue out=w1508:refnum<queue>, error out=w1507:errorcluster)  [unwired: 1 in, 1 out]
        }
        frame 7 {
          # "DATALOG OF OP 40"
          n560 = Enqueue Element(queue=w1515, element=cluster{"CASE 2":T12} {"CASE 2"=enum."DATALOG4"}, error in (no error)=w1514) -> (queue out=w1513:refnum<queue>, error out=w1512:errorcluster)  [unwired: 1 in, 1 out]
        }
        frame 8 {
          # "SCAN BARCODE OP 50"
          n561 = Enqueue Element(queue=w1520, element=cluster{"CASE":T12} {"CASE"=enum."SCAN5"}, error in (no error)=w1519) -> (queue out=w1518:refnum<queue>, error out=w1517:errorcluster)  [unwired: 1 in, 1 out]
        }
        frame 9 {
          # "DATALOG OF OP 50"
          n562 = Enqueue Element(queue=w1525, element=cluster{"CASE":T12} {"CASE"=enum."DATALOG5"}, error in (no error)=w1524) -> (queue out=w1523:refnum<queue>, error out=w1522:errorcluster)  [unwired: 1 in, 1 out]
        }
        frame 10 {
          # "SCAN BARCODE OP 60"
          n563 = Enqueue Element(queue=w1530, element=cluster{"CASE 2":T12} {"CASE 2"=enum."SCAN6"}, error in (no error)=w1529) -> (queue out=w1528:refnum<queue>, error out=w1527:errorcluster)  [unwired: 1 in, 1 out]
        }
        frame 11 {
          # "DATALOG OF OP 60"
          n564 = Enqueue Element(queue=w1535, element=cluster{"CASE 2":T12} {"CASE 2"=enum."DATALOG6"}, error in (no error)=w1534) -> (queue out=w1533:refnum<queue>, error out=w1532:errorcluster)  [unwired: 1 in, 1 out]
        }
        frame 12 {
          # "SCAN BARCODE OP 70"
          n565 = Enqueue Element(queue=w1540, element=cluster{"CASE 2":T12} {"CASE 2"=enum."SCAN7"}, error in (no error)=w1539) -> (queue out=w1538:refnum<queue>, error out=w1537:errorcluster)  [unwired: 1 in, 1 out]
        }
        frame 13 {
          # "DATALOG OF OP 70"
          n566 = Enqueue Element(queue=w1545, element=cluster{"CASE 2":T12} {"CASE 2"=enum."DATALOG7"}, error in (no error)=w1544) -> (queue out=w1543:refnum<queue>, error out=w1542:errorcluster)  [unwired: 1 in, 1 out]
        }
        frame 14 {
          # "SCAN BARCODE 80"
          n567 = Enqueue Element(queue=w1550, element=cluster{"CASE 2":T12} {"CASE 2"=enum."SCAN8"}, error in (no error)=w1549) -> (queue out=w1548:refnum<queue>, error out=w1547:errorcluster)  [unwired: 1 in, 1 out]
        }
        frame 15 {
          # "DATALOG OF OP 80"
          n568 = Enqueue Element(queue=w1555, element=cluster{"CASE 2":T12} {"CASE 2"=enum."DATALOG8"}, error in (no error)=w1554) -> (queue out=w1553:refnum<queue>, error out=w1552:errorcluster)  [unwired: 1 in, 1 out]
        }
        frame 16 {
          # "SCAN BARCODE OP 90"
          n569 = Enqueue Element(queue=w1560, element=cluster{"CASE 2":T12} {"CASE 2"=enum."SCAN9"}, error in (no error)=w1559) -> (queue out=w1558:refnum<queue>, error out=w1557:errorcluster)  [unwired: 1 in, 1 out]
        }
        frame 17 {
          # "DATALOG OF OP 90"
          n570 = Enqueue Element(queue=w1565, element=cluster{"CASE 2":T12} {"CASE 2"=enum."DATALOG9"}, error in (no error)=w1564) -> (queue out=w1563:refnum<queue>, error out=w1562:errorcluster)  [unwired: 1 in, 1 out]
        }
        frame 18 {
          # "SCAN BARCODE OP 100"
          n571 = Enqueue Element(queue=w1570, element=cluster{"CASE 2":T12} {"CASE 2"=enum."SCAN10"}, error in (no error)=w1569) -> (queue out=w1568:refnum<queue>, error out=w1567:errorcluster)  [unwired: 1 in, 1 out]
        }
        frame 19 {
          # "DATALOG OF OP 100"
          n572 = Enqueue Element(queue=w1575, element=cluster{"CASE 2":T12} {"CASE 2"=enum."DATALOG10"}, error in (no error)=w1574) -> (queue out=w1573:refnum<queue>, error out=w1572:errorcluster)  [unwired: 1 in, 1 out]
        }
        frame 20 {
          # "SCAN BARCODE OP 110"
          n573 = Enqueue Element(queue=w1580, element=cluster{"CASE 2":T12} {"CASE 2"=enum."SCAN11"}, error in (no error)=w1579) -> (queue out=w1578:refnum<queue>, error out=w1577:errorcluster)  [unwired: 1 in, 1 out]
        }
        frame 21 {
          # "DATALOG OF OP 110"
          n574 = Enqueue Element(queue=w1585, element=cluster{"CASE 2":T12} {"CASE 2"=enum."DATALOG11"}, error in (no error)=w1584) -> (queue out=w1583:refnum<queue>, error out=w1582:errorcluster)  [unwired: 1 in, 1 out]
        }
      }
    }
    n575 = Wait (ms)(milliseconds to wait=u32 50) -> ()  [unwired: 1 out]
    n576 = global read "Global 1.vi" "PLC COMM"() -> (→"PLC COM.":bool)
    n577 = global read "Global 1.vi" "PLC 1"() -> (→"OP 10 & 20":bool)
    n578 = global read "Global 1.vi" "PLC 2"() -> (→"OP 30":bool)
    n579 = global read "Global 1.vi" "PLC 3"() -> (→"OP 40":bool)
    n580 = case shown="False" "stop 2" {
      tunnel: w1424 -> [w1434 w1440]
      tunnel: [w1434 w1439] -> w1422
      tunnel: w1423 -> [w1433 w1438]
      tunnel: [w1433 w1437] -> w1421
      tunnel: [FALSE TRUE] -> w1420
      frame False {
      }
      frame True {
        n581 = Flush Queue(queue=w1440, error in (no error)=w1438) -> (queue out=w1442:refnum<queue>, error out=w1441:errorcluster)  [unwired: 1 out]
        n582 = Enqueue Element(queue=w1442, element=cluster{"CASE 2":T12} {"CASE 2"=enum."STOP"}, error in (no error)=w1441) -> (queue out=w1439:refnum<queue>, error out=w1437:errorcluster)  [unwired: 1 in, 1 out]
      }
    }
    "stop" <- w1420
    n583 = global read "Global 1.vi" "PLC 4"() -> (→"OP 50":bool)
    n584 = global read "Global 1.vi" "PLC 5"() -> (→"OP 60":bool)
    n585 = global read "Global 1.vi" "PLC 7"() -> (→"OP 90 -100 - 110":bool)
    n586 = global read "Global 1.vi" "PLC 6"() -> (→"OP 70 & 80":bool)
  }
  n587 = Release Queue(queue=w66, error in (no error)=w72) -> (error out=w49:errorcluster)  [unwired: 1 in, 2 out]
  n588 = call <vilib>:"Clear Errors.vi"("error in (no error)"=w68) -> ("error out"=w53:errorcluster)  [unwired: 5 in, 1 out]
  n589 = call <vilib>:"DB Tools Close Connection.vi"("error in (no error)"=w53, "connection reference"=w67) -> ("error out"=w50:errorcluster)  [unwired: 5 in]
  n590 = Merge Errors(w49, w50) -> (w51:errorcluster)
  n591 = call <vilib>:"Simple Error Handler.vi"("error in (no error)"=w51) -> ("error out"=w46:errorcluster)  [unwired: 4 in, 4 out]
  n592 = call <vilib>:"Clear Errors.vi"("error in (no error)"=w46) -> ("error out"=w52:errorcluster)  [unwired: 5 in, 1 out]
  n593 = flat-sequence {
    tunnel: w52 -> [w1588]
    tunnel: [w1588] -> w54
    frame #0 {
      n594 = global write "Global 1.vi" "REMOVE VI"(TRUE ("remove_VI")) -> ()
      n595 = global write "DATA LOG.vi" "Auto Cycle On"(FALSE) -> ()
    }
  }
  n596 = property class="App"(error in=w54) -> (error out=w56:errorcluster, "App.Kind"=w55:T36)  [unwired: 1 in, 1 out]
  n597 = case shown="\"Run Time System\"" w55 {
    tunnel: [w1589 w1591] -> w57
    tunnel: w56 -> [w1589 w1590]
    frame "Development System", Default {
    }
    frame "Run Time System" {
      n598 = invoke class="VI" method="FP.Close"(error in=w1590) -> (error out=w1591:errorcluster)  [unwired: 2 in, 2 out]
    }
  }
  "error out 2" <- w57
